vi "Dashboard Main.vi"() -> ()   [LabVIEW 2015]
uses:
  Vision FRC Color Processing Example Folder - Copy/Vision Support Code/Camera Types.ctl
  <vilib>/Utility/miscctls.llb/LVRowAndColumnTypeDef.ctl
  <vilib>/event_ctls.llb/eventvkey.ctl
  <vilib>/Rock Robotics/Network Tables/NT Write Boolean.vi
  <vilib>/Rock Robotics/Network Tables/NT Read Boolean.vi
  <vilib>/Rock Robotics/WPI/Dashboard/WPI_DashboardLogging Global.vi
  <vilib>/Utility/config.llb/Write Key (String).vi
  <vilib>/Utility/config.llb/Write Key (I32).vi
  <vilib>/Rock Robotics/Network Tables/NT Read Numeric Array.vi
  <vilib>/Utility/config.llb/NI_LVConfig.lvlib
panel:
  in  "Camera Type":T1=enum."1011"
  in  "TCP":refnum<k5>
  in  "Rec Mode":enum32{"Stop", "Record", "Playback"}(radio)
  in  "Vision":u16(ring) items=["Camera Off", "USB Camera SW", "USB Camera HW", "IP Camera"]
  out "Camera IP":string
  out "Image Message":string="Timeout in Camera Communications"
  in  "Dashboard Tab":T2(tab)=enum."Custom"
  out "Shooter Current":dbl(slide) scale=0.0..40.0
  out "Angle At Setpoint":bool=TRUE
  in  "Shoot":bool
  in  "Defense Type":T3(ring)
  out "NT Connection":bool
  in  "Camera Settings":T4={"Frame Rate"=30, "Compression"=30, "Size"=1} {"Frame Rate" scale=1.0..30.0; "Size" items=["640x480", "320x240", "160x120"]}
  out "Mode":T5(ring)=enum."Auto Disabled"
  in  "DB Camera Config":bool
  out "fps":dbl format="%#.1g"
  out "Mbps":dbl format="%#.1g"
  out "Mbps LED":bool
  out "Arm Encoder":dbl(slide) scale=-1.0..1.0
  out "At Target":bool
  in  "Defense Location":enum16{"0", "1", "2", "3", "4", "5"}(ring)
  in  "DB/String 0":string
  in  "DB/Slider 1":dbl(slide) scale=0.0..5.0
  out "DB/LED 1":bool
  out "DB/LED 0":bool
  in  "DB/Button 3":bool
  in  "DB/Button 2":bool
  in  "DB/Button 1":bool caption="LED Light"
  in  "DB/Button 0":bool
  out "JS1 Z":dbl(slide) scale=-1.0..1.0 scale format="%#_2e"
  out "JS1 Graph":cluster{"X":dbl, "Y":dbl}[](graph)
  out "JS1 Buttons":T6
  out "JS2 Z":dbl(slide) scale=-1.0..1.0 scale format="%#_2e"
  out "JS2 Graph":cluster{"X":dbl, "Y":dbl}[](graph)
  out "JS2 Buttons":T6
  out "Shooter Current":dbl(graph)
  out "Detected Targets":T7(array[cluster]) {"Normalized Rect"."Numeric 5" format="%#_2g"; "Normalized Rect"."Numeric 3" format="%#_2g"; "Normalized Rect"."Numeric 2" format="%#_2g"; "Normalized Rect"."Numeric" format="%#_2g"}
  in  "LED Color":T8={"Hue"={85.0, 140.0}, "Sat"={190.0, 255.0}, "Val"={70.0, 255.0}} {"Hue" scale=0.0..255.0 scale format="%#_3g"}
  in  "Std Devs for Calibration":cluster{"H":dbl, "S":dbl, "V":dbl}={"H"=4.0, "S"=6.0, "V"=6.0}
  in  "Min Score Threshold":i32=70
  out "Target Distance":dbl
  out "Target X":dbl
  out "Target Y":dbl
  in  "Test Slider":dbl(slide) scale=0.0..100.0 scale format="%#_3g"
  in  "On/Off":bool caption="Solenoid"
  in  "Test Name":u16(ring) items=["Select the test to run..."]
  in  "Test Tree":string(tree)
  in  "Motor":cluster{"Value":dbl, "Enable":bool} {"Value" scale=-1.0..1.0 scale format="%#_3g"}
  out "Progress":T9 {"Test Progress" scale=0.0..100.0}
  in  "Rev/Fwd":cluster{"Forward":bool, "Reverse":bool}
  in  "Test Ring":u16(ring) items=["Monochrome", "Color"]
  out "Cmd Status":string
  in  "Execute Command":bool
  in  "Command Params":string[][](table)
  in  "Command Selection":i32(listbox)
  in  "CheckList":i32(listbox)
  out "Tree":string(tree)
  out "Camera Image":T10(plugin-control)
  out "Background":bool
  # "Right"
  # "Left"
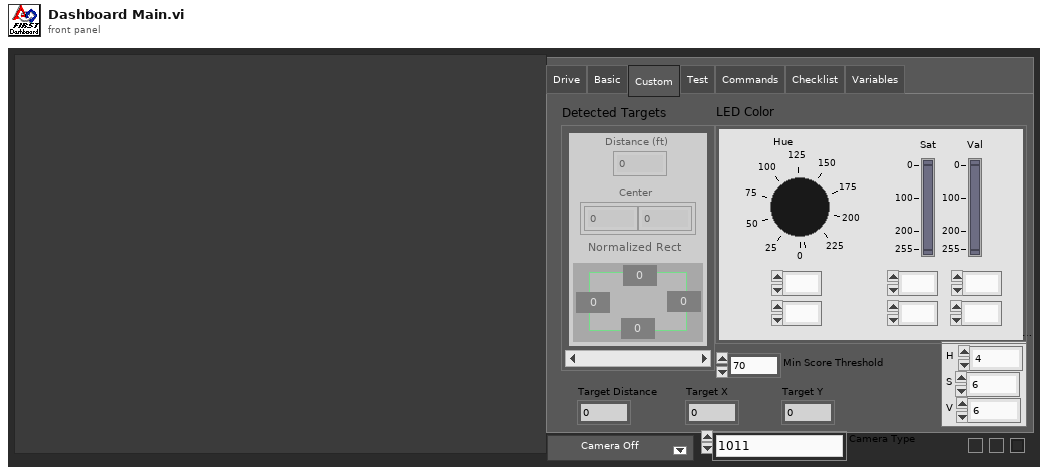
[diagram p1: front panel]
types:
  T1 = typedef "Camera Types.ctl" = enum16{"206", "1011", "1013", "MS HD3000 square", "MS HD3000 640x480"}
  T2 = enum32{"Drive", "Basic", "Custom", "Test", "Commands", "Checklist", "Variables"}
  T3 = enum16{"None", "Rampart", "Moat", "Rock Wall", "Rough Terrain", "Low Bar", "Chili Fries"}
  T4 = cluster{"Frame Rate":i32, "Compression":i32, "Size":u16}
  T5 = enum8{"Tele-Op Disabled", "Tele-Op Enabled", "Auto Disabled", "Auto Enabled", "Test Disabled", "Test Enabled", "Disconnected", "No Code", "E-Stop"}
  T6 = cluster{bool, bool, bool, bool, bool, bool, bool, bool, bool, bool, bool, bool}
  T7 = cluster{"Distance (ft)":dbl, "Center":cluster{dbl, dbl}, "Normalized Rect":cluster{"Numeric":dbl, "Numeric 2":dbl, "Numeric 3":dbl, "Numeric 5":dbl}}[]
  T8 = cluster{"Hue":cluster{dbl, dbl}, "Sat":cluster{dbl, dbl}, "Val":cluster{dbl, dbl}}
  T9 = cluster{"Test Progress":u8, "Test Progress Text":string}
  T10 = typedef "IMAQ Image.ctl" = refnum<image>
  T11 = cluster{"IDs":cluster{"RPC field ID":u16, "Unique ID":u16}, "String":string}
  T12 = enum32{"Drive", "Basic", "Custom", "Test", "Checklist", "Variables"}
  T13 = typedef "Image Type" = u32
  T14 = cluster{"Detected Targets[0]":cluster{"Distance (ft)":dbl, "Center":cluster{dbl, dbl}, "Normalized Rect":cluster{"Numeric":dbl, "Numeric 2":dbl, "Numeric 3":dbl, "Numeric 5":dbl}}, "Detected Targets[1]":cluster{"Distance (ft)":dbl, "Center":cluster{dbl, dbl}, "Normalized Rect":cluster{"Numeric":dbl, "Numeric 2":dbl, "Numeric 3":dbl, "Numeric 5":dbl}}, "Detected Targets[2]":cluster{"Distance (ft)":dbl, "Center":cluster{dbl, dbl}, "Normalized Rect":cluster{"Numeric":dbl, "Numeric 2":dbl, "Numeric 3":dbl, "Numeric 5":dbl}}, "Detected Targets[3]":cluster{"Distance (ft)":dbl, "Center":cluster{dbl, dbl}, "Normalized Rect":cluster{"Numeric":dbl, "Numeric 2":dbl, "Numeric 3":dbl, "Numeric 5":dbl}}, "Detected Targets[4]":cluster{"Distance (ft)":dbl, "Center":cluster{dbl, dbl}, "Normalized Rect":cluster{"Numeric":dbl, "Numeric 2":dbl, "Numeric 3":dbl, "Numeric 5":dbl}}, "Detected Targets[5]":cluster{"Distance (ft)":dbl, "Center":cluster{dbl, dbl}, "Normalized Rect":cluster{"Numeric":dbl, "Numeric 2":dbl, "Numeric 3":dbl, "Numeric 5":dbl}}, "Detected Targets[6]":cluster{"Distance (ft)":dbl, "Center":cluster{dbl, dbl}, "Normalized Rect":cluster{"Numeric":dbl, "Numeric 2":dbl, "Numeric 3":dbl, "Numeric 5":dbl}}, "Detected Targets[7]":cluster{"Distance (ft)":dbl, "Center":cluster{dbl, dbl}, "Normalized Rect":cluster{"Numeric":dbl, "Numeric 2":dbl, "Numeric 3":dbl, "Numeric 5":dbl}}, "Detected Targets[8]":cluster{"Distance (ft)":dbl, "Center":cluster{dbl, dbl}, "Normalized Rect":cluster{"Numeric":dbl, "Numeric 2":dbl, "Numeric 3":dbl, "Numeric 5":dbl}}}
  T15 = cluster{"Distance (ft)":dbl, "Center":cluster{dbl, dbl}, "Normalized Rect":cluster{"Numeric":dbl, "Numeric 2":dbl, "Numeric 3":dbl, "Numeric 5":dbl}}
  T16 = cluster{"Numeric":dbl, "Numeric 2":dbl, "Numeric 3":dbl, "Numeric 5":dbl}
  T17 = cluster{"Camera Image":refnum<vi>, "Dashboard Tab":refnum<vi>, "Background":refnum<vi>, "Vision":refnum<vi>, "Rec Mode":refnum<vi>, "Test Slider":refnum<vi>, "On/Off ":refnum<vi>, "Test Ring":refnum<vi>, "Rev/Fwd":refnum<vi>, "Test Name":refnum<vi>, "Motor":refnum<vi>, "Progress":refnum<vi>, "CheckList":refnum<vi>, "Tree":refnum<vi>, "Test Tree":refnum<vi>, "Command Params":refnum<vi>, "Command Selection":refnum<vi>, "Execute Command":refnum<vi>, "Cmd Status":refnum<vi>}
  T18 = typedef "NI_LVConfig.lvlib/Config Data RefNum.ctl" = refnum<k1>
  T19 = cluster{"Operation":enum16{"Update", "Clear"}, "Color Box":u32}[]
  T20 = typedef "eventvkey.ctl" = enum16{"ASCII", "Enter", "Return", "Shift", "Ctrl", "Alt", "Cmd", "Opt", "Caps", "NumLock", "Clear", "Break", "Up", "Down", "Left", "Right", "Insert", "Delete", "Home", "End", "PageUp", "PageDown", "Escape", "Help", "Pause", "ScrollLock", "F1", "F2", "F3", "F4", "F5", "F6", "F7", "F8", "F9", "F10", "F11", "F12", "F13", "F14", "F15", "F16", "F17", "F18", "F19", "F20", "F21", "F22", "F23", "F24", "Play", "VolumeUp", "VolumeDown", "Mute", "Two Byte Char"}
  T21 = cluster{"Image Size":bool, "Image Type":bool, "Pixel Value":bool, "ROI Information":bool, "Zoom Factor":bool}
  T22 = enum8{"Enabled", "Disabled", "Disabled and Grayed Out"}
  T23 = cluster{"Operation":enum16{"Update", "Clear"}, "Color Box":u32}
  T24 = typedef "LVRowAndColumnTypeDef.ctl" = cluster{"Row":i32, "Column":i32}
  T25 = cluster{"Shift":bool, "Ctrl":bool, "Alt":bool, "Cmd":bool, "Opt":bool}
  T26 = enum16{"open", "open or create", "create or replace", "create", "open (read only)"}
  T27 = cluster{"Error Strings":string, "Disable Counts":cluster{u16, u16}, "Rail Faults":cluster{u16, u16, u16}, "Robot IP":string, "DB Mode":u8, "Event Info":cluster{"Name":string, "Type":u8, "Number":u16, "Replay":u8}, "Camera Addr":string}
  T28 = cluster{"Storage":cluster{"Disk Free":u64, "RAM Block":u32, "RAM free":u32}, "CPU Utilization":cluster{"CPU % ISR":sgl, "CPU % Time Crit":sgl, "CPU % Timed Str":sgl, "CPU % High":sgl, "CPU % Above":sgl, "CPU % Normal":sgl, "CPU % Low":sgl}, "CAN":cluster{"% Bus Utilization":sgl, "Bus Off Cnt":u32, "TX_FIFO Full Cnt":u32, "Receive Error Cnt":u8, "Transmit Error Cnt":u8}, "HID":cluster{"HID Outputs":u32, "Rumble Low":u16, "Rumble High":u16}[]}
  T29 = cluster{"Status bits":cluster{"Test Mode":bool, "Autonomous":bool, "Enabled":bool, "Code Start":bool, "Brownout":bool, "Reserved 2":bool, "Reserved 3":bool, "E-Stop":bool}, "Code Trace":cluster{"Disabled":bool, "TeleOp":bool, "Auto":bool, "Test":bool}, "Controller Type":enum16{"unknown", "cRIO", "roboRio"}, "Code?":enum16{"unknown", "noCode", "code"}, "Battery V":dbl}
  T30 = cluster{"Control Bits":cluster{"TestMode":bool, "Autonomous":bool, "Enabled":bool, "FMS Present":bool, bool, bool, bool, "E-Stop":bool}, "Team Station ":u8, "Countdown":sgl, "Joystick Values":cluster{"Axes":dbl[], "Buttons":bool[], "POVs":i16[]}[]}
  T31 = cluster{"Axes":dbl[], "Buttons":bool[], "POVs":i16[]}[]
  T32 = cluster{"Test Mode":bool, "Autonomous":bool, "Enabled":bool, "Code Start":bool, "Brownout":bool, "Reserved 2":bool, "Reserved 3":bool, "E-Stop":bool}
  T33 = cluster{"Axes":dbl[], "Buttons":bool[], "POVs":i16[]}
  T34 = cluster{"Buttons[0]":bool, "Buttons[1]":bool, "Buttons[2]":bool, "Buttons[3]":bool, "Buttons[4]":bool, "Buttons[5]":bool, "Buttons[6]":bool, "Buttons[7]":bool, "Buttons[8]":bool, "Buttons[9]":bool, "Buttons[10]":bool, "Buttons[11]":bool}
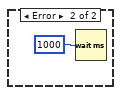
[diagram p2: hidden frame]
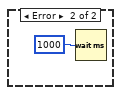
[diagram p3: hidden frame]
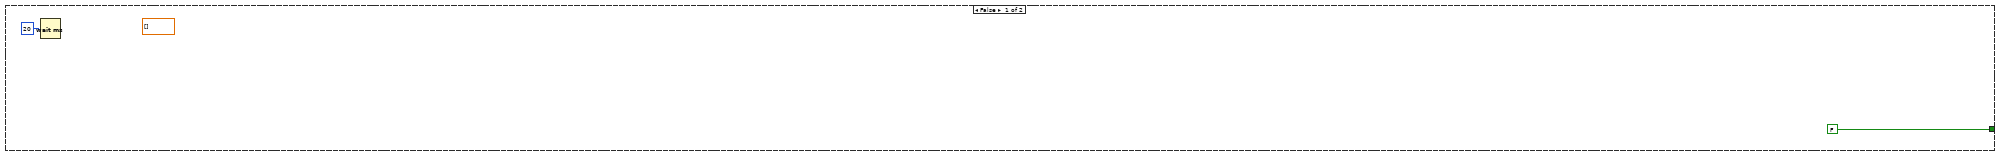
[diagram p4: hidden frame]
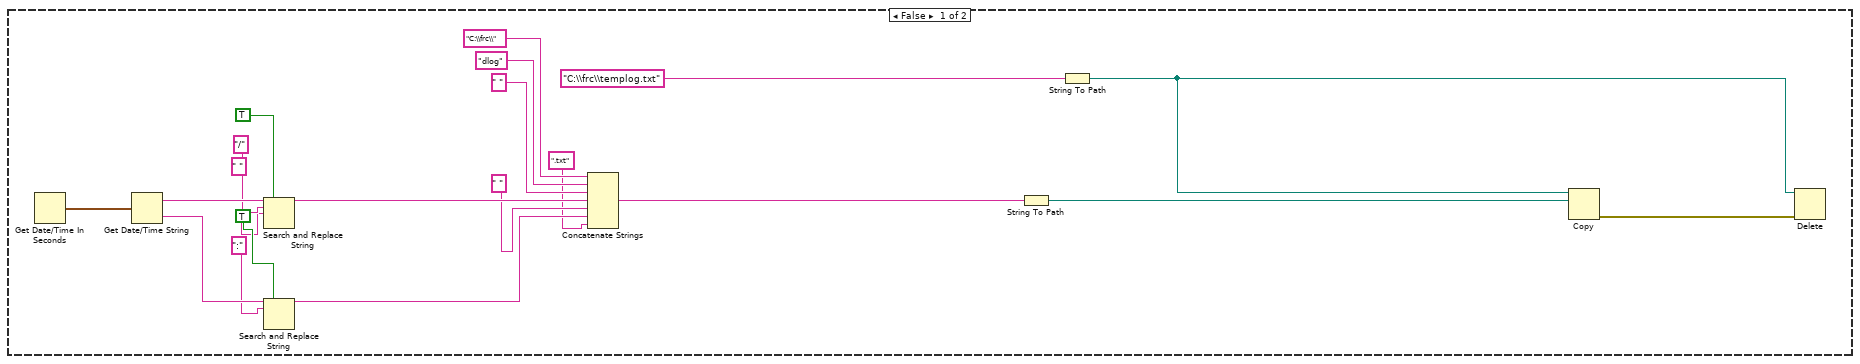
[diagram p5: hidden frame]
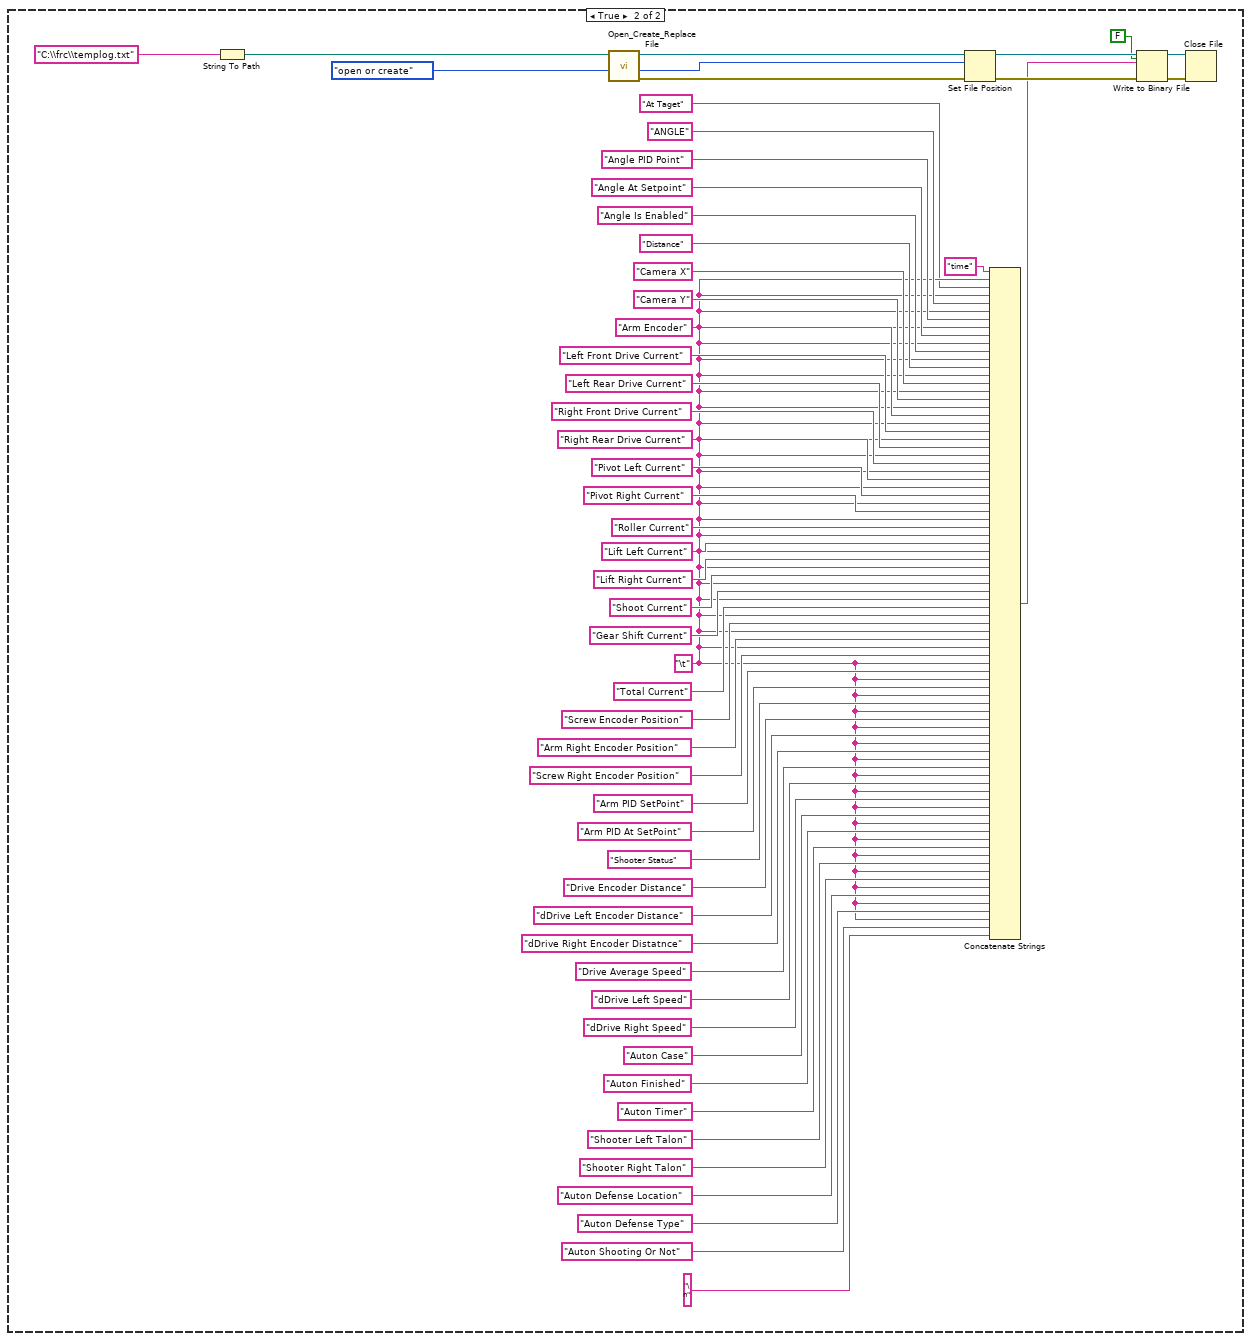
[diagram p6: hidden frame]
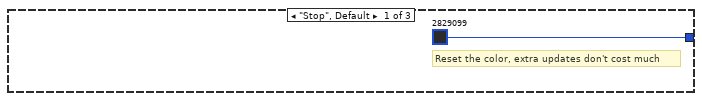
[diagram p7: hidden frame]
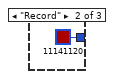
[diagram p8: hidden frame]
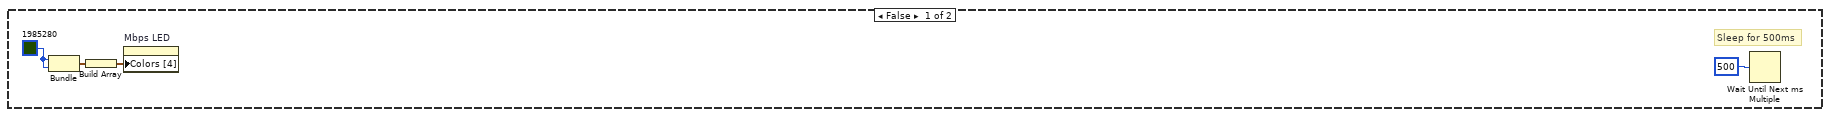
[diagram p10: hidden frame]
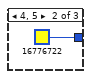
[diagram p11: hidden frame]
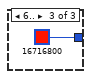
[diagram p12: hidden frame]
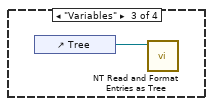
[diagram p14: hidden frame]
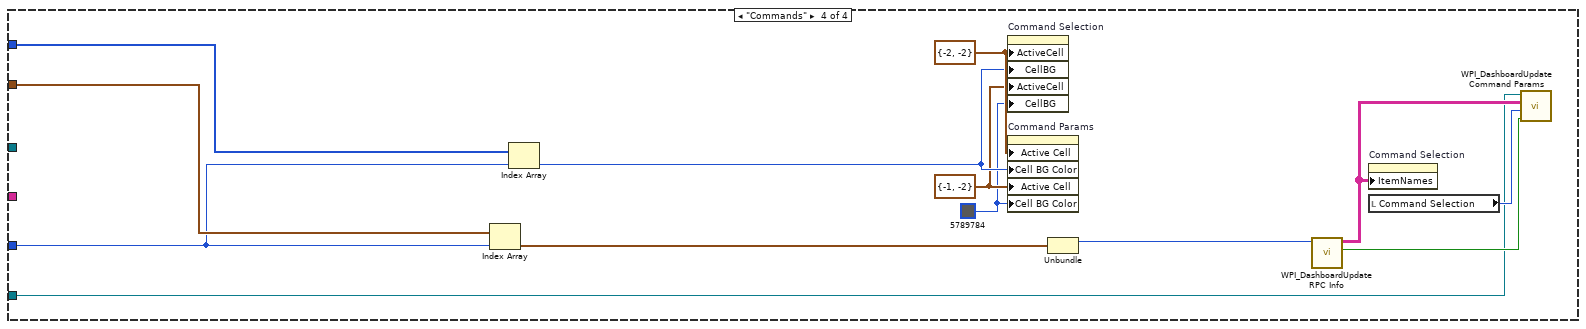
[diagram p15: hidden frame]
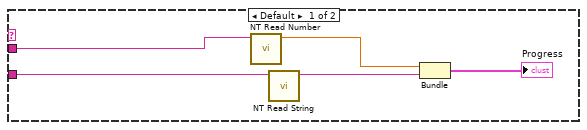
[diagram p16: hidden frame]
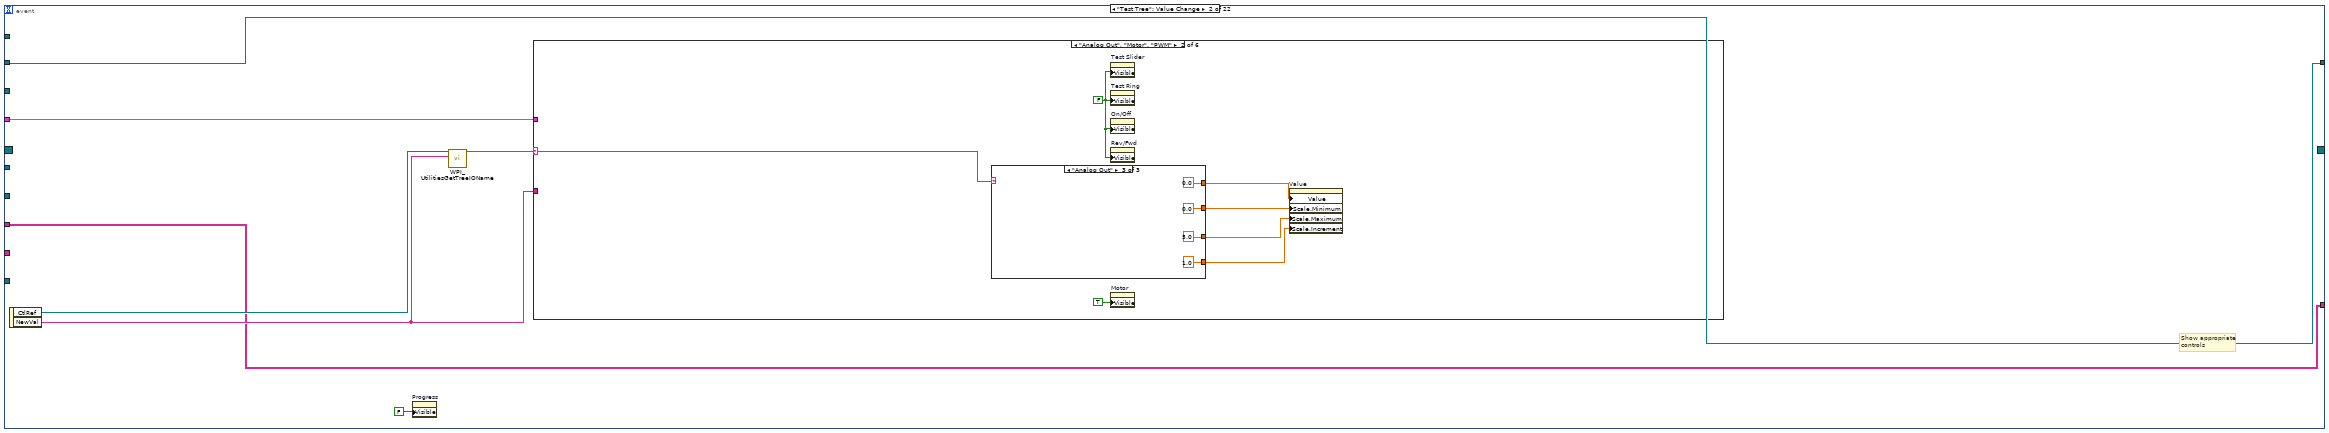
[diagram p17: hidden frame]
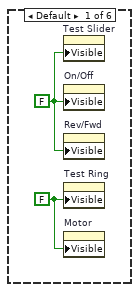
[diagram p18: hidden frame]
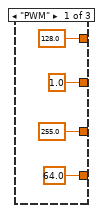
[diagram p19: hidden frame]
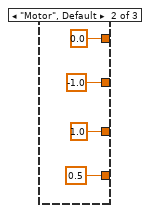
[diagram p20: hidden frame]
diagram:
  w10 = T11 {"IDs"={"RPC field ID"=0, "Unique ID"=0}, "String"=""}  # RPC Response
  w34 = 491  # min tab size
  w33 = 1.333  # min tab size
  w42 = enum32{"Stop", "Record", "Playback"}."Stop" ("Rec Mode")
  w16 = FALSE ("Visible")
  (unwired) "This VI has seven parallel loops for different tasks and a bit of initialization code that runs just once.\n\nTypical dashboard extensions only need to edit the panel. Adding new indicators or controls simply involves placing them on the panel in the Operations tab and naming them the same as the SmartDashboard variable on the robot\n\nIf the display needs to process the data before display, loop one is an example of doing that for the joysticks and motors.\n\nIf you want customize the video display or perform processing on it, loop two is where that takes place.\n\nOther loops should not need to be modified. They are pretty standard, and document the task they perform."  # Documentation
  w62 = T13 4 items=["Grayscale (U8)", "Grayscale (I16)", "Grayscale (SGL)", "Complex (CSG)", "RGB (U32)", "HSL (U32)", "RGB (U64)"] ("Image Type")
  # "Loop 7. Wait for DS connections"
  # "Controls for Test Mode, Camera Settings, etc."
  # "Loop 6. Animation for background of window during playback and record"
  # "Fires each time robot IP\nchanges, simulator does this"
  # "Fires each time window\ndocking changes."
  # "Collects all controls and indicators\nin the Basic and Custom tab.\nIf you need to bind additional controls,\nadd their references. You can extend the\nenum constant or use an integer."
  # "Loop 4. Process UI events related to test mode, checklist, and camera settings"
  # "Loop 3. Wait until the robot response provides\n the Robot IP address.\nOnce known, bind controls and\nvariables with the same names."
  # "Loop 5. Adjusts placement onscreen, hides the titlebar, etc."
  # "Loop 1. Receive various data streams from Driver Station, update joystick, motors, and more complex displays that don't easily bind to variables."
  # "Loop 2. Receive camera images from Robot, update Mbps, fps, and do any processing or display"
  n1 = control-ref of="Dashboard Tab"() -> (w40:refnum<vi>)
  n2 = property class="VI"() -> ("Panel"=w49:refnum<vi>)  [unwired: 2 in, 2 out]
  n3 = property on="Camera Settings" class="Clust (strict)"("Visible"=w16) -> ()  [unwired: 2 in, 2 out]
  n4 = property on="On/Off" class="Bool (strict)"("Visible"=w16) -> ()  [unwired: 2 in, 2 out]
  n5 = property on="Rev/Fwd" class="Clust (strict)"("Visible"=w16) -> ()  [unwired: 2 in, 2 out]
  n6 = local write "DB Camera Config"(w16) -> ()
  n7 = property on="Motor" class="Clust (strict)"("Visible"=w16) -> ()  [unwired: 2 in, 2 out]
  n8 = property on="Progress" class="Clust (strict)"("Visible"=w16) -> ()  [unwired: 2 in, 2 out]
  n9 = property on="Test Ring" class="Ring (strict)"("Visible"=w16) -> ()  [unwired: 2 in, 2 out]
  n10 = local write "Command Selection"(u16 0 ("milliseconds to wait")) -> ()
  n11 = local write "Rec Mode"(w42) -> ()
  n12 = global write "WPI_DashboardLogging Global.vi" "Recording"(w42) -> ()
  n13 = property class="Pnl"(reference=w49) -> ("Panes[]"=w50:refnum<vi>[])  [unwired: 1 in, 2 out]
  n14 = local write "Command Params"(string[][] [] ("Command Params")) -> ()
  n15 = local write "Dashboard Tab"(T2."Drive" ("Dashboard Tab")) -> ()
  n16 = call "IMAQ Create"("Image Name"="Dashboard Image", "Image Type"=w62) -> ("New Image"=w60:T10, "error out"=w59:errorcluster)  [unwired: 2 in, 1 out]
  n17 = Index Array(array=w50) -> (element=w48:refnum<vi>)  [unwired: 1 in]
  n18 = while {
    tunnel: w60 -> [w80]
    tunnel: w59 -> [_]
    tunnel: [w81] -> _
    i -> [w81]
    stop <- FALSE stop-if-true
    # "Optionally read the DB image,\nlog, or retrieve images from a\nlogged match"
    n19 = local read "Shooter Current"() -> (→"Shooter Current":dbl)
    n20 = call-poly <vilib>:"NT Write Value.vi"("Numeric"="Defense Type", "Name"="Defense Type") -> ()  [unwired: 9 in, 1 out]
    n21 = call-poly <vilib>:"NT Write Value.vi"("Numeric"="Defense Location", "Name"="Defense Location") -> ()  [unwired: 9 in, 1 out]
    n22 = call-poly <vilib>:"NT Read Value.vi"("Name"="Angle At Setpoint") -> ("Boolean"=→"Angle At Setpoint":bool)  [unwired: 9 in, 1 out]
    n23 = call-poly <vilib>:"NT Write Value.vi"("Boolean"="Shoot", "Name"="Shoot") -> ()  [unwired: 9 in, 1 out]
    n24 = local read "Camera IP"() -> (w74:string)
    n25 = local read "Rec Mode"() -> (w75:enum32{"Stop", "Record", "Playback"})
    n26 = call <vilib>:"WPI_CameraRead MJPG for Dashboard.vi"("Camera Settings"="Camera Settings", "Rec Mode"=w75, "Camera IP"=w74, "Camera Mode"="Vision", "Refnum in"=w80) -> ("Active"=w78:bool, "Refnum out"=w79:T10, "FPS"=w77:dbl, "Bandwidth (Mbps)"=w73:dbl)  [unwired: 3 in]
    "Mbps" <- w73
    n27 = case shown="True" w78 {
      tunnel: w79 -> [_ w177]
      tunnel: w73 -> [_ w176]
      tunnel: w77 -> [_ w175]
      frame False {
        w83 = u32 1985280 ("Color Box")
        # "Sleep for 500ms"
        n28 = Bundle("Color Box"=w83, "Color Box"=w83) -> (w85:cluster{"Color Box":u32, "Color Box":u32})  [unwired: 1 out]
        n29 = Build Array(w85) -> (w84:cluster{"Color Box":u32, "Color Box":u32}[])
        n30 = property on="Mbps LED" class="Bool (strict)"("Colors [4]"=w84) -> ()  [unwired: 2 in, 2 out]
        n31 = Wait Until Next ms Multiple(millisecond multiple=u32 500) -> ()  [unwired: 1 out]
      }
      frame True {
        # "Here is where you would annotate,\npossibly process, and display the image"
        # "Update Mbps LED"
        n32 = case shown="Default" w176 {
          tunnel: [u32 6618880 ("Color Box") u32 16776722 ("Color Box") u32 16716800 ("Color Box")] -> w178
          frame Default {
          }
          frame 4, 5 {
          }
          frame 6.. {
          }
        }
        n33 = call "IMAQ Clear Overlay"("Image"=w177) -> ("error out"=w181:errorcluster, "Image Out"=w174:T10)  [unwired: 2 in, 7 out]
        n34 = Unbundle By Name(w181) -> ("status"=w182:bool)
        n35 = call "FRC Color Processing Example.vi"("Std Devs for Calibration"="Std Devs for Calibration", "LED Color"="LED Color", "Min Score Threshold"="Min Score Threshold", "New Image"=w174, "Camera Type"="Camera Type") -> ("Detected Targets"=w131:T7, "Original Image"=→"Camera Image":T10)  [unwired: 5 in]
        "Detected Targets" <- w131
        n36 = property on="Image Message" class="Str"("Visible"=w182) -> ()  [unwired: 2 in, 2 out]
        n37 = Bundle("Color Box"=w178, "Color Box"=w178) -> (w180:cluster{"Color Box":u32, "Color Box":u32})  [unwired: 1 out]
        n38 = Array To Cluster(array=w131) -> (cluster=w169:T14)
        n39 = Build Array(w180) -> (w179:cluster{"Color Box":u32, "Color Box":u32}[])
        n40 = property on="Mbps LED" class="Bool (strict)"("Colors [4]"=w179) -> ()  [unwired: 2 in, 2 out]
        n41 = Unbundle(w169) -> ("Detected Targets[0]"=w168:T15, "Detected Targets[1]"=w144:T15, "Detected Targets[2]"=w132:T15)  [unwired: 6 out]
        n42 = Unbundle(w168) -> ("Distance (ft)"=w105:dbl, "Center"=w167:cluster{dbl, dbl}, "Normalized Rect"=w166:T16)
        n43 = Unbundle(w144) -> ("Distance (ft)"=w100:dbl, "Center"=w145:cluster{dbl, dbl}, "Normalized Rect"=w146:T16)
        n44 = Unbundle(w132) -> ("Distance (ft)"=w94:dbl, "Center"=w143:cluster{dbl, dbl}, "Normalized Rect"=w142:T16)
        n45 = Not Equal To 0?(x=w105) -> (x != 0?=w108:bool)
        n46 = Not Equal To 0?(x=w100) -> (x != 0?=w103:bool)
        n47 = Not Equal To 0?(x=w94) -> (x != 0?=w97:bool)
        n48 = Unbundle(w167) -> (w126:dbl)  [unwired: 1 out]
        n49 = Unbundle(w166) -> ("Numeric"=w158:dbl, "Numeric 2"=w125:dbl, "Numeric 3"=w156:dbl, "Numeric 5"=w160:dbl)
        n50 = Unbundle(w145) -> (w130:dbl)  [unwired: 1 out]
        n51 = Unbundle(w146) -> ("Numeric"=w153:dbl, "Numeric 2"=w124:dbl, "Numeric 3"=w155:dbl, "Numeric 5"=w151:dbl)
        n52 = Unbundle(w143) -> (w129:dbl)  [unwired: 1 out]
        n53 = Unbundle(w142) -> ("Numeric"=w135:dbl, "Numeric 2"=w123:dbl, "Numeric 3"=w133:dbl, "Numeric 5"=w137:dbl)
        n54 = Build Array(w126, w130, w129) -> (w127:dbl[])
        n55 = Build Array(w125, w124, w123) -> (w122:dbl[])
        n56 = Select(t=w105, s=w108, f=100.0) -> (s? t:f=w104:dbl)
        n57 = Select(t=w100, s=w103, f=100.0) -> (s? t:f=w99:dbl)
        n58 = Select(t=w94, s=w97, f=100.0) -> (s? t:f=w95:dbl)
        n59 = call-poly <vilib>:"NT Write Value.vi"("Numeric"=w126, "Name"="ImageXCenter0") -> ()  [unwired: 9 in, 1 out]
        n60 = call-poly <vilib>:"NT Write Value.vi"("Numeric"=w158, "Name"="ImageLeft0") -> ()  [unwired: 9 in, 1 out]
        n61 = call-poly <vilib>:"NT Write Value.vi"("Numeric"=w125, "Name"="ImageTop0") -> ()  [unwired: 9 in, 1 out]
        n62 = call-poly <vilib>:"NT Write Value.vi"("Numeric"=w156, "Name"="ImageRight0") -> ()  [unwired: 9 in, 1 out]
        n63 = call-poly <vilib>:"NT Write Value.vi"("Numeric"=w160, "Name"="ImageBottom0") -> ()  [unwired: 9 in, 1 out]
        n64 = call-poly <vilib>:"NT Write Value.vi"("Numeric"=w130, "Name"="ImageXCenter1") -> ()  [unwired: 9 in, 1 out]
        n65 = call-poly <vilib>:"NT Write Value.vi"("Numeric"=w153, "Name"="ImageLeft1") -> ()  [unwired: 9 in, 1 out]
        n66 = call-poly <vilib>:"NT Write Value.vi"("Numeric"=w124, "Name"="ImageTop1") -> ()  [unwired: 9 in, 1 out]
        n67 = call-poly <vilib>:"NT Write Value.vi"("Numeric"=w155, "Name"="ImageRight1") -> ()  [unwired: 9 in, 1 out]
        n68 = call-poly <vilib>:"NT Write Value.vi"("Numeric"=w151, "Name"="ImageBottom1") -> ()  [unwired: 9 in, 1 out]
        n69 = call-poly <vilib>:"NT Write Value.vi"("Numeric"=w129, "Name"="ImageXCenter2") -> ()  [unwired: 9 in, 1 out]
        n70 = call-poly <vilib>:"NT Write Value.vi"("Numeric"=w135, "Name"="ImageLeft2") -> ()  [unwired: 9 in, 1 out]
        n71 = call-poly <vilib>:"NT Write Value.vi"("Numeric"=w123, "Name"="ImageTop2") -> ()  [unwired: 9 in, 1 out]
        n72 = call-poly <vilib>:"NT Write Value.vi"("Numeric"=w133, "Name"="ImageRight2") -> ()  [unwired: 9 in, 1 out]
        n73 = call-poly <vilib>:"NT Write Value.vi"("Numeric"=w137, "Name"="ImageBottom2") -> ()  [unwired: 9 in, 1 out]
        n74 = Multiply(x=1.142, y=w104) -> (x*y=w110:dbl)
        n75 = Multiply(x=1.142, y=w99) -> (x*y=w116:dbl)
        n76 = Multiply(x=1.142, y=w95) -> (x*y=w113:dbl)
        n77 = Subtract(x=w110, y=1.0255) -> (x-y=w106:dbl)
        n78 = Subtract(x=w116, y=1.0255) -> (x-y=w101:dbl)
        n79 = Subtract(x=w113, y=1.0255) -> (x-y=w98:dbl)
        n80 = Build Array(w106, w101, w98) -> (w128:dbl[])
        n81 = call-poly <vilib>:"NT Write Value.vi"("Numeric"=w106, "Name"="distanceToTarget0") -> ()  [unwired: 9 in, 1 out]
        n82 = call-poly <vilib>:"NT Write Value.vi"("Numeric"=w101, "Name"="distanceToTarget1") -> ()  [unwired: 9 in, 1 out]
        n83 = call-poly <vilib>:"NT Write Value.vi"("Numeric"=w98, "Name"="distanceToTarget2") -> ()  [unwired: 9 in, 1 out]
        n84 = Array Max & Min(array=w128) -> (min value=w89:dbl, min index (indices)=w121:i32)  [unwired: 2 out]
        "Target Distance" <- w89
        n85 = Index Array(array=w127, index=w121) -> (element=w120:dbl)
        "Target X" <- w120
        n86 = Index Array(array=w122, index=w121) -> (element=→"Target Y":dbl)
        n87 = In Range and Coerce(upper limit=-0.1525, x=w120, lower limit=-0.1725) -> (In Range?=w91:bool)  [unwired: 1 out]
        n88 = Less?(x=w89, y=15.0) -> (x < y?=w90:bool)
        n89 = And(x=w91, y=w90) -> (x .and. y?=w88:bool)
        "At Target" <- w88
        n90 = call-poly <vilib>:"NT Write Value.vi"("Boolean"=w88, "Name"="At Target") -> ()  [unwired: 9 in, 1 out]
        "fps" <- w175
      }
    }
  }
  n91 = while {
    tunnel: u16 1741 ("timeout ms (25000)") -> [w187]
    stop <- FALSE stop-if-true
    n92 = TCP Create Listener(10:w187) -> (0:w186:errorcluster, 3:w188:refnum<k5>)  [unwired: 4 in, 1 out]
    n93 = case shown="No Error" w186 {
      selector: w186 -> [w190 _]
      tunnel: w188 -> [w191 _]
      frame No Error {
        n94 = while {
          tunnel: w191 -> [w194]
          tunnel: w190 -> [w193]
          stop <- FALSE stop-if-true
          n95 = TCP Wait On Listener(8:w193, 11:w194) -> (0:w195:errorcluster, 4:w196:refnum<k5>)  [unwired: 2 in, 3 out]
          n96 = case shown="No Error" w195 {
            frame No Error {
            }
            frame Error {
              n97 = Wait (ms)(milliseconds to wait=u32 1000) -> ()  [unwired: 1 out]
            }
          }
          n98 = local write "TCP"(w196) -> ()
        }
      }
      frame Error {
        n99 = Wait (ms)(milliseconds to wait=u32 1000) -> ()  [unwired: 1 out]
      }
    }
  }
  n100 = call <vilib>:"Get Tab Control Refs.vi"("Page Index"=T12."Custom" ("Dashboard Tab"), "TabControl in"=w40) -> ("ControlsOnPage"=w39:refnum<vi>[])  [unwired: 9 in]
  n101 = while {
    tunnel: w48 -> [w200]
    i -> [w203]
    stop <- FALSE stop-if-true
    n102 = case shown="\"Playback\"" "Rec Mode" {
      tunnel: w203 -> [_ _ w218]
      tunnel: [u32 2829099 ("Base Color") u32 11141120 ("Target Color") w207] -> w199
      frame "Stop", Default {
        # "Reset the color, extra updates don't cost much"
      }
      frame "Record" {
      }
      frame "Playback" {
        # "Playback"
        n103 = Quotient & Remainder(x=w218, y=u32 50 ("milliseconds to wait")) -> (x-y*floor(x/y)=w214:u32)  [unwired: 1 out]
        n104 = Divide(x=w214, y=u32 50 ("milliseconds to wait")) -> (x/y=w211:dbl)
        n105 = Multiply(x=6.283185307179586, y=w211) -> (x*y=w216:dbl)
        n106 = Sine(x=w216) -> (sin(x)=w215:dbl)
        n107 = Absolute Value(x=w215) -> (abs(x)=w208:dbl)
        n108 = call "Interpolate RGB Color.vi"("Proportion"=w208, "Target Color"=u32 30976, "Base Color"=u32 2829099) -> ("Result Color"=w207:u32)  [unwired: 8 in]
      }
    }
    n109 = Wait (ms)(milliseconds to wait=u32 100) -> ()  [unwired: 1 out]
    n110 = property class="Pane"(reference=w200, "PaneColor"=w199) -> ()  [unwired: 1 in, 2 out]
  }
  n111 = call <vilib>:"Get Tab Control Refs.vi"("Page Index"=T12."Basic" ("Dashboard Tab"), "TabControl in"=w40) -> ("ControlsOnPage"=w15:refnum<vi>[])  [unwired: 9 in]
  n112 = Build Array (concatenate)(w15, w39) -> (w38:refnum<vi>[])
  n113 = Obtain Notifier(name (unnamed)="Robot IP Update", notification data type="IP Addr" ("name (unnamed)")) -> (notifier out=w2:refnum<notifier>)  [unwired: 2 in, 2 out]
  n114 = Create User Event(user event datatype=w10) -> (user event=w6:refnum<user-event>)  [unwired: 1 in, 1 out]
  n115 = control-ref of="Rec Mode"() -> (w22:refnum<vi>)
  n116 = control-ref of="Command Selection"() -> (w9:refnum<vi>)
  n117 = control-ref of="Execute Command"() -> (w11:refnum<vi>)
  n118 = control-ref of="Command Params"() -> (w12:refnum<vi>)
  n119 = control-ref of="Camera Image"() -> (w37:refnum<vi>)
  n120 = control-ref of="Dashboard Tab"() -> (w36:refnum<vi>)
  n121 = control-ref of="Tree"() -> (w26:refnum<vi>)
  n122 = control-ref of="Test Tree"() -> (w25:refnum<vi>)
  n123 = control-ref of="Background"() -> (w31:refnum<vi>)
  n124 = control-ref of="Cmd Status"() -> (w5:refnum<vi>)
  n125 = control-ref of="On/Off"() -> (w20:refnum<vi>)
  n126 = control-ref of="Test Name"() -> (w24:refnum<vi>)
  n127 = control-ref of="Test Slider"() -> (w21:refnum<vi>)
  n128 = control-ref of="Rev/Fwd"() -> (w18:refnum<vi>)
  n129 = control-ref of="Motor"() -> (w23:refnum<vi>)
  n130 = control-ref of="Progress"() -> (w17:refnum<vi>)
  n131 = control-ref of="CheckList"() -> (w27:refnum<vi>)
  n132 = control-ref of="Test Ring"() -> (w19:refnum<vi>)
  n133 = control-ref of="Vision"() -> (w35:refnum<vi>)
  n134 = while {
    tunnel: w38 -> [w231]
    tunnel: w2 -> [w229]
    tunnel: [w227] -> _
    tunnel: u32 1000 ("milliseconds to wait") -> [w226]
    tunnel: w6 -> [w219]
    i -> [w227]
    stop <- FALSE stop-if-true
    n135 = Wait on Notification(notifier=w229, timeout in ms (-1)=w226) -> (notification=w228:string, timed out?=w224:bool)  [unwired: 2 in, 2 out]
    n136 = local read "Rec Mode"() -> (w222:enum32{"Stop", "Record", "Playback"})
    n137 = Equal?(x=w222, y=u16 2 ("Rec Mode")) -> (x = y?=w223:bool)
    n138 = Compound Arithmetic op=OR(invert w224, w223) -> (w225:bool)
    n139 = case shown="True" w225 {
      tunnel: w231 -> [_ w235]
      tunnel: w228 -> [_ w234]
      tunnel: "Dashboard" -> [_ w233]
      tunnel: w219 -> [_ w232]
      frame False {
      }
      frame True {
        n140 = call <vilib>:"Bind Controls to SmartDashboard.vi"("RPC ref"=w232, "Client Name"=w233, "Bound Control Refs"=w235, "Server IP Address"=w234) -> ()  [unwired: 8 in]
      }
    }
  }
  n141 = Bundle("Camera Image"=w37, "Dashboard Tab"=w36, "Background"=w31, "Vision"=w35, "Rec Mode"=w22, "Test Slider"=w21, "On/Off"=w20, "Test Ring"=w19, "Rev/Fwd"=w18, "Test Name"=w24, "Motor"=w23, "Progress"=w17, "CheckList"=w27, "Tree"=w26, "Test Tree"=w25, "Command Params"=w12, "Command Selection"=w9, "Execute Command"=w11, "Cmd Status"=w5) -> (w28:T17)  [unwired: 1 in]
  n142 = register-events(refnum<vi> refnum, w6) -> (reference out=w46:refnum<event-registration>, error out=w45:errorcluster)  [unwired: 2 in]
  n143 = call "Initialize Camera and CheckList.vi"("ListBox in"=w27) -> ("Cluster"=w53:cluster{"value":i32, "value":i32, "index":i32}, "Array"=w54:cluster{string[]}[], "File Refnum"=w52:T18)  [unwired: 8 in]
  n144 = property on="Camera Settings" class="Clust (strict)"("Val(Sgnl)"=w53) -> ()  [unwired: 2 in, 2 out]
  n145 = Bundle("min tab size"=w34, "min tab size"=w33) -> (w32:cluster{"min tab size":i32, "min tab size":dbl})  [unwired: 1 in]
  n146 = Obtain Notifier(name (unnamed)="Window Mode", notification data type=TRUE) -> (notifier out=w3:refnum<notifier>)  [unwired: 2 in, 2 out]
  n147 = vi-ref "Playback Controls.vi"() -> (w47:refnum<vi>)
  n148 = control-ref of="Command Params"() -> (w4:refnum<vi>)
  n149 = control-ref of="Test Tree"() -> (w51:refnum<vi>)
  n150 = property class="VI" props=["Front Panel.Closeable"]() -> (reference out=w41:refnum<vi>)  [unwired: 2 in, 2 out]
  n151 = call "Adjust Dashboard Window.vi"("Sizing Refnums"=w28, "Size Constraints"=w32, "VI"=w41, "WIn Mode"=w3) -> ()  [unwired: 8 in]
  n152 = while {
    tunnel: w54 -> [w247]
    shift-right: [w246] -> _
    shift-left: w52 -> [w245]
    tunnel: [w244] -> _
    tunnel: w51 -> [w243]
    tunnel: w47 -> [w242]
    tunnel: w46 -> [w241]
    tunnel: w45 -> [_]
    tunnel: w41 -> [w240]
    tunnel: w6 -> [w239]
    tunnel: w4 -> [w238]
    shift-right: [w237] -> _
    shift-left: _ -> [w236]
    i -> [w244]
    stop <- FALSE stop-if-true
    n153 = event shown="[0] Timeout" {
      selector: w241 -> [_ _ _ _ _ _ _ _ _ _ _ _ _ _ _ _ _ _ _ _ _ _]
      dyn-events: [_ _ _ _ _ _ _ _ _ _ _ _ _ _ _ _ w548 _ _ _ _ _] -> _
      timeout: u32 60 ("milliseconds to wait") -> [_ _ _ _ _ _ _ _ _ _ _ _ _ _ _ _ _ _ _ _ _ _]
      tunnel: w243 -> [w260 _ _ _ _ _ _ _ _ _ _ _ _ _ _ _ _ _ _ _ _ _]
      tunnel: "Test Tree" -> [_ _ _ _ _ _ _ _ _ _ _ w511 w520 w523 w528 w537 _ _ _ _ _ _]
      tunnel: w247 -> [_ w298 _ _ _ _ _ _ _ w473 w504 _ _ _ _ _ _ _ _ _ _ _]
      tunnel: [w257 w297 w401 w407 w419 w431 w439 w445 w458 w472 w497 w510 w518 w522 w527 w536 w550 w566 w568 w576 w587 w592] -> w246
      tunnel: w245 -> [w257 w297 w401 w407 w419 w431 w439 w445 w458 w471 w497 w510 w518 w522 w527 w536 w550 w566 w568 w576 w587 w592]
      tunnel: w242 -> [_ _ _ _ _ _ _ _ _ _ _ _ _ _ _ _ w551 _ w571 _ _ _]
      tunnel: w240 -> [_ _ _ _ _ _ _ _ _ _ _ _ _ _ _ _ w546 _ _ _ _ _]
      tunnel: w239 -> [_ _ _ _ _ _ _ _ _ _ _ _ _ _ _ _ w542 _ _ _ _ _]
      tunnel: w238 -> [w252 _ _ _ w417 _ _ _ _ _ _ _ _ _ _ _ _ _ _ _ _ _]
      tunnel: [w251 w296 w400 w406 w415 w425 w436 w444 w457 w470 w496 w509 w517 w521 w526 w535 w541 w564 w567 w572 w580 w593] -> w237
      tunnel: w236 -> [w251 w296 w400 w406 w415 _ _ w444 w457 w470 w496 w509 w517 w521 w526 w535 w541 w564 w567 w572 w580 w593]
      event Timeout {
        n154 = event-data() -> ()  [unwired: 1 in, 1 out]
        n155 = local read "Mode"() -> (w254:T5)
        n156 = call <vilib>:"Connextion Info.vi"() -> ("Connected"=→"NT Connection":bool)  [unwired: 10 in, 1 out]
        n157 = case shown="\"Test\"" "Dashboard Tab" {
          tunnel: w260 -> [_ w274 _ _]
          tunnel: "/TestMode/Automatic/" ("Name Pattern") -> [_ w273 _ _]
          tunnel: T19 [{"Operation"=enum."Clear", "Color Box"=14013909}, {"Operation"=enum."Clear", "Color Box"=14013909}, {"Operation"=enum."Clear", "Color Box"=14013909}, {"Operation"=enum."Clear", "Color Box"=14013909}, {"Operation"=enum."Update", "Color Box"=14013909}, {"Operation"=enum."Update", "Color Box"=16777215}, {"Operation"=enum."Clear", "Color Box"=14013909}, {"Operation"=enum."Clear", "Color Box"=14013909}, {"Operation"=enum."Clear", "Color Box"=14013909}] -> [_ w266 _ w283]
          tunnel: w254 -> [_ w265 _ w282]
          tunnel: u32[] [15790320, 15790320, 15790320, 15790320, 16777215, 16777215, 15790320, 15790320, 15790320] -> [_ _ _ w288]
          tunnel: w252 -> [_ _ _ w276]
          frame "Custom", Default {
          }
          frame "Test" {
            w272 = -2 ("Active Item:Row Number")
            n158 = Index Array(array=w266, index=w265) -> (element=w267:T23)
            n159 = Unbundle(w267) -> ("Operation"=w268:enum16{"Update", "Clear"}, "Color Box"=w269:u32)
            n160 = call <vilib>:"NT Read and Format Entries as Tree.vi"("Operation"=w268, "Name Pattern"=w273, "Tree Refnum"=w274) -> ()  [unwired: 7 in, 2 out]
            n161 = property on="Test Tree" class="Tree (strict)"("Active Item Row Number"=w272, "ActiveColNum"=w272, "CellBG"=w269, "Active Item Row Number"=-1 ("Active Item:Row Number"), "CellBG"=u32 5789784 ("Color Box")) -> ()  [unwired: 2 in, 2 out]
          }
          frame "Variables" {
            n162 = control-ref of="Tree"() -> (w275:refnum<vi>)
            n163 = call <vilib>:"NT Read and Format Entries as Tree.vi"("Tree Refnum"=w275) -> ()  [unwired: 9 in, 2 out]
          }
          frame "Commands" {
            w284 = u32 5789784 ("Color Box")
            w285 = T24 {"Row"=-1, "Column"=-2} ("Active Cell:Active Cell")
            w287 = T24 {"Row"=-2, "Column"=-2} ("Active Cell:Active Cell")
            n164 = Index Array(array=w283, index=w282) -> (element=w281:T23)
            n165 = Index Array(array=w288, index=w282) -> (element=w286:u32)
            n166 = property on="Command Selection" class="MCListbox (strict)"("ActiveCell"=w287, "CellBG"=w286, "ActiveCell"=w285, "CellBG"=w284) -> ()  [unwired: 2 in, 2 out]
            n167 = property on="Command Params" class="Tbl (strict)"("Active Cell"=w287, "Cell BG Color"=w286, "Active Cell"=w285, "Cell BG Color"=w284) -> ()  [unwired: 2 in, 2 out]
            n168 = Unbundle(w281) -> ("Operation"=w280:enum16{"Update", "Clear"})  [unwired: 1 out]
            n169 = call <vilib>:"WPI_DashboardUpdate RPC Info.vi"("Operation"=w280) -> ("update"=w278:bool, "commands"=w277:string[][])  [unwired: 9 in]
            n170 = property on="Command Selection" class="MCListbox (strict)"("ItemNames"=w277) -> ()  [unwired: 2 in, 2 out]
            n171 = local read "Command Selection"() -> (w279:i32)
            n172 = call <vilib>:"WPI_DashboardUpdate Command Params.vi"("Update"=w278, "NewVal"=w279, "Commands"=w277, "Param Tbl"=w276) -> ()  [unwired: 7 in, 1 out]
          }
        }
        n173 = call <vilib>:"NT Read String.vi"("Name"="/TestMode/TestName") -> ("String"=w263:string)  [unwired: 9 in, 1 out]
        n174 = case shown="\"\"" w263 {
          tunnel: "/TestMode/TestProgress" ("Name") -> [w290 _]
          tunnel: "/TestMode/TestProgressText" ("Name") -> [w289 _]
          frame Default {
            n175 = call <vilib>:"NT Read Number.vi"("Name"=w290) -> ("Numeric"=w291:dbl)  [unwired: 9 in, 1 out]
            n176 = call <vilib>:"NT Read String.vi"("Name"=w289) -> ("String"=w292:string)  [unwired: 9 in, 1 out]
            n177 = Bundle("Numeric"=w291, "String"=w292) -> (→"Progress":cluster{"Numeric":dbl, "String":string})  [unwired: 1 in]
          }
          frame "" {
            n178 = property on="Progress" class="Clust (strict)"("Visible"=FALSE) -> ()  [unwired: 2 in, 2 out]
            n179 = local write "Test Name"(u16 0) -> ()
          }
        }
      }
      event "Test Tree": Value Change {
        # "Show appropriate\ncontrols"
        n180 = event-data() -> ("CtlRef"=w301:refnum<vi>, "NewVal"=w299:string)  [unwired: 1 in]
        n181 = property on="Progress" class="Clust (strict)"("Visible"=FALSE) -> ()  [unwired: 2 in, 2 out]
        n182 = call <vilib>:"WPI_UtilitiesGetTreeIOName.vi"("NewVal"=w299, "TreeControl in"=w301) -> ("I/O Name"=w302:string)  [unwired: 9 in]
        n183 = case shown="\"Analog Out\", \"Motor\", \"PWM\"" w302 {
          selector: w302 -> [_ w309 _ w331 w340 _]
          tunnel: w299 -> [_ _ w328 w330 _ w347]
          tunnel: w298 -> [_ _ _ _ _ w346]
          frame Default {
            w304 = FALSE ("Visible")
            w303 = FALSE ("Visible")
            n184 = property on="Test Slider" class="Slide (strict)"("Visible"=w304) -> ()  [unwired: 2 in, 2 out]
            n185 = property on="On/Off" class="Bool (strict)"("Visible"=w304) -> ()  [unwired: 2 in, 2 out]
            n186 = property on="Rev/Fwd" class="Clust (strict)"("Visible"=w304) -> ()  [unwired: 2 in, 2 out]
            n187 = property on="Test Ring" class="Ring (strict)"("Visible"=w303) -> ()  [unwired: 2 in, 2 out]
            n188 = property on="Motor" class="Clust (strict)"("Visible"=w303) -> ()  [unwired: 2 in, 2 out]
          }
          frame "Analog Out", "Motor", "PWM" {
            w310 = FALSE ("Visible")
            n189 = case shown="\"Analog Out\"" w309 {
              tunnel: [1.0 ("Value") -1.0 ("Value") 0.0 ("Value")] -> w308
              tunnel: [255.0 ("Value") 1.0 ("Value") 5.0 ("Value")] -> w307
              tunnel: [128.0 ("Value") 0.0 ("Value") 0.0 ("Value")] -> w306
              tunnel: [64.0 ("Value") 0.5 ("Value") 1.0 ("Value")] -> w305
              frame "PWM" {
              }
              frame "Motor", Default {
              }
              frame "Analog Out" {
              }
            }
            n190 = property on="Test Slider" class="Slide (strict)"("Visible"=w310) -> ()  [unwired: 2 in, 2 out]
            n191 = property on="Test Ring" class="Ring (strict)"("Visible"=w310) -> ()  [unwired: 2 in, 2 out]
            n192 = property on="On/Off" class="Bool (strict)"("Visible"=w310) -> ()  [unwired: 2 in, 2 out]
            n193 = property on="Rev/Fwd" class="Clust (strict)"("Visible"=w310) -> ()  [unwired: 2 in, 2 out]
            n194 = property on="Motor" class="Clust (strict)"("Visible"=TRUE) -> ()  [unwired: 2 in, 2 out]
            n195 = property on="Value" class="Slide (strict)"("Value"=w306, "Scale.Minimum"=w308, "Scale.Maximum"=w307, "Scale.Increment"=w305) -> ()  [unwired: 2 in, 2 out]
          }
          frame "Servo" {
            w326 = FALSE ("Visible")
            n196 = call <vilib>:"NT Read Number.vi"("Name"=w328) -> ("Numeric"=w327:dbl)  [unwired: 9 in, 1 out]
            n197 = property on="Motor" class="Clust (strict)"("Visible"=w326) -> ()  [unwired: 2 in, 2 out]
            n198 = property on="Test Ring" class="Ring (strict)"("Visible"=w326) -> ()  [unwired: 2 in, 2 out]
            n199 = property on="On/Off" class="Bool (strict)"("Visible"=w326) -> ()  [unwired: 2 in, 2 out]
            n200 = property on="Rev/Fwd" class="Clust (strict)"("Visible"=w326) -> ()  [unwired: 2 in, 2 out]
            n201 = property on="Test Slider" class="Slide (strict)"("Visible"=TRUE, "Scale.Maximum"=170.0 ("Scale.Range:Maximum")) -> ()  [unwired: 2 in, 2 out]
            n202 = local write "Test Slider"(w327) -> ()
          }
          frame "Relay", "Solenoid" {
            w329 = FALSE ("Visible")
            n203 = property on="Motor" class="Clust (strict)"("Visible"=w329) -> ()  [unwired: 2 in, 2 out]
            n204 = property on="Test Slider" class="Slide (strict)"("Visible"=w329) -> ()  [unwired: 2 in, 2 out]
            n205 = property on="Test Ring" class="Ring (strict)"("Visible"=w329) -> ()  [unwired: 2 in, 2 out]
            n206 = Search and Replace String(input string=w330, search string="/Value  **", replace string="/Direction") -> (result string=w336:string)  [unwired: 5 in, 3 out]
            n207 = call <vilib>:"NT Read String.vi"("Name"=w336) -> ("String"=w334:string)  [unwired: 9 in, 1 out]
            n208 = Equal?(x="Both directions", y=w334) -> (x = y?=w332:bool)
            n209 = property on="Rev/Fwd" class="Clust (strict)"("Visible"=w332) -> ()  [unwired: 2 in, 2 out]
            n210 = Not(x=w332) -> (.not. x?=w333:bool)
            n211 = property on="On/Off" class="Bool (strict)"("Visible"=w333, "Caption.Text"=w331) -> ()  [unwired: 2 in, 2 out]
          }
          frame "Compressor", "Digital Out" {
            w339 = FALSE ("Visible")
            # "Get direction and finish"
            n212 = property on="Test Ring" class="Ring (strict)"("Visible"=w339) -> ()  [unwired: 2 in, 2 out]
            n213 = property on="Motor" class="Clust (strict)"("Visible"=w339) -> ()  [unwired: 2 in, 2 out]
            n214 = property on="Test Slider" class="Slide (strict)"("Visible"=w339) -> ()  [unwired: 2 in, 2 out]
            n215 = property on="Rev/Fwd" class="Clust (strict)"("Visible"=FALSE) -> ()  [unwired: 2 in, 2 out]
            n216 = property on="On/Off" class="Bool (strict)"("Visible"=TRUE, "Caption.Text"=w340) -> ()  [unwired: 2 in, 2 out]
          }
          frame "Camera" {
            n217 = call <vilib>:"Get Last Path Segment.vi"("String in"=w347) -> ("String out"=w348:string)  [unwired: 10 in]
            n218 = property on="Rev/Fwd" class="Clust (strict)"("Visible"=FALSE) -> ()  [unwired: 2 in, 2 out]
            n219 = case shown="\"White Balance  **\"" w348 {
              tunnel: w347 -> [w354 w363 w372 w381 w390 _ w396]
              tunnel: w346 -> [w352 w360 w369 w378 w387 _ _]
              frame "Size  **" {
                n220 = Index Array(array=w352) -> (element=w351:cluster{string[]})  [unwired: 1 in]
                n221 = call <vilib>:"NT Read String.vi"("Name"=w354) -> ("String"=w353:string)  [unwired: 9 in, 1 out]
                n222 = property on="Test Ring" class="Ring (strict)"("Visible"=TRUE) -> ()  [unwired: 2 in, 2 out]
                n223 = property on="Test Slider" class="Slide (strict)"("Visible"=FALSE) -> ()  [unwired: 2 in, 2 out]
                n224 = Unbundle(w351) -> (w349:string[])
                n225 = Match First String(2:w349, 3:w353) -> (0:w350:i32)  [unwired: 1 out]
                n226 = property on="Test Ring" class="Ring (strict)"("Value"=w350, "Strings []"=w349) -> ()  [unwired: 2 in, 2 out]
              }
              frame "White Balance  **" {
                n227 = call <vilib>:"NT Read String.vi"("Name"=w363) -> ("String"=w362:string)  [unwired: 9 in, 1 out]
                n228 = Index Array(array=w360, index=1) -> (element=w361:cluster{string[]})
                n229 = property on="Test Ring" class="Ring (strict)"("Visible"=TRUE) -> ()  [unwired: 2 in, 2 out]
                n230 = property on="Test Slider" class="Slide (strict)"("Visible"=FALSE) -> ()  [unwired: 2 in, 2 out]
                n231 = Unbundle(w361) -> (w358:string[])
                n232 = Match First String(2:w358, 3:w362) -> (0:w357:i32)  [unwired: 1 out]
                n233 = property on="Test Ring" class="Ring (strict)"("Value"=w357, "Strings []"=w358) -> ()  [unwired: 2 in, 2 out]
              }
              frame "Exposure  **" {
                n234 = call <vilib>:"NT Read String.vi"("Name"=w372) -> ("String"=w371:string)  [unwired: 9 in, 1 out]
                n235 = Index Array(array=w369, index=2) -> (element=w370:cluster{string[]})
                n236 = property on="Test Ring" class="Ring (strict)"("Visible"=TRUE) -> ()  [unwired: 2 in, 2 out]
                n237 = property on="Test Slider" class="Slide (strict)"("Visible"=FALSE) -> ()  [unwired: 2 in, 2 out]
                n238 = Unbundle(w370) -> (w366:string[])
                n239 = Match First String(2:w366, 3:w371) -> (0:w367:i32)  [unwired: 1 out]
                n240 = property on="Test Ring" class="Ring (strict)"("Value"=w367, "Strings []"=w366) -> ()  [unwired: 2 in, 2 out]
              }
              frame "Exposure Priority  **" {
                n241 = call <vilib>:"NT Read String.vi"("Name"=w381) -> ("String"=w380:string)  [unwired: 9 in, 1 out]
                n242 = Index Array(array=w378, index=3) -> (element=w379:cluster{string[]})
                n243 = property on="Test Ring" class="Ring (strict)"("Visible"=TRUE) -> ()  [unwired: 2 in, 2 out]
                n244 = property on="Test Slider" class="Slide (strict)"("Visible"=FALSE) -> ()  [unwired: 2 in, 2 out]
                n245 = Unbundle(w379) -> (w375:string[])
                n246 = Match First String(2:w375, 3:w380) -> (0:w376:i32)  [unwired: 1 out]
                n247 = property on="Test Ring" class="Ring (strict)"("Value"=w376, "Strings []"=w375) -> ()  [unwired: 2 in, 2 out]
              }
              frame "Color Enable  **" {
                n248 = call <vilib>:"NT Read String.vi"("Name"=w390) -> ("String"=w389:string)  [unwired: 9 in, 1 out]
                n249 = Index Array(array=w387, index=4) -> (element=w388:cluster{string[]})
                n250 = property on="Test Ring" class="Ring (strict)"("Visible"=TRUE) -> ()  [unwired: 2 in, 2 out]
                n251 = property on="Test Slider" class="Slide (strict)"("Visible"=FALSE) -> ()  [unwired: 2 in, 2 out]
                n252 = Unbundle(w388) -> (w384:string[])
                n253 = Match First String(2:w384, 3:w389) -> (0:w385:i32)  [unwired: 1 out]
                n254 = property on="Test Ring" class="Ring (strict)"("Value"=w385, "Strings []"=w384) -> ()  [unwired: 2 in, 2 out]
              }
              frame Default {
                n255 = property on="Test Slider" class="Slide (strict)"("Visible"=FALSE) -> ()  [unwired: 2 in, 2 out]
                n256 = property on="Test Ring" class="Ring (strict)"("Visible"=FALSE) -> ()  [unwired: 2 in, 2 out]
              }
              frame "Brightness  **", "Color Level  **", "Compression  **", "FPS  **", "Sharpness  **" {
                n257 = call <vilib>:"NT Read Number.vi"("Name"=w396) -> ("Numeric"=w395:dbl)  [unwired: 9 in, 1 out]
                n258 = property on="Test Ring" class="Ring (strict)"("Visible"=FALSE) -> ()  [unwired: 2 in, 2 out]
                n259 = property on="Test Slider" class="Slide (strict)"("Visible"=TRUE, "Scale.Maximum"=100.0 ("Scale.Range:Maximum")) -> ()  [unwired: 2 in, 2 out]
                n260 = local write "Test Slider"(w395) -> ()
              }
            }
            n261 = property on="Motor" class="Clust (strict)"("Visible"=FALSE) -> ()  [unwired: 2 in, 2 out]
            n262 = property on="On/Off" class="Bool (strict)"("Visible"=FALSE) -> ()  [unwired: 2 in, 2 out]
          }
        }
      }
      event "Test Name": Mouse Enter {
        # "Populate the ring with the list of tests"
        n263 = event-data() -> ()  [unwired: 1 in, 1 out]
        n264 = call <vilib>:"NT Read String Array.vi"("Name"="/TestMode/TestList") -> ("String Array"=w405:string[])  [unwired: 9 in, 1 out]
        n265 = Build Array (concatenate)("Select the test to run...", w405) -> (w404:string[])
        n266 = property on="Test Name" class="Ring (strict)"("Strings []"=w404) -> ()  [unwired: 2 in, 2 out]
      }
      event "Test Name": Value Change {
        w408 = FALSE ("Visible")
        # "Tell the robot the test name to run"
        n267 = event-data() -> ("NewVal"=w412:u16)  [unwired: 1 in]
        n268 = property on="Test Name" class="Ring (strict)"() -> ("Strings []"=w413:string[])  [unwired: 2 in, 2 out]
        n269 = Index Array(array=w413, index=w412) -> (element=w411:string)
        n270 = local write "Progress"(T9 {"Test Progress"=0, "Test Progress Text"=""} ("Progress")) -> ()
        n271 = property on="Progress" class="Clust (strict)"("Visible"=TRUE) -> ()  [unwired: 2 in, 2 out]
        n272 = property on="Test Ring" class="Ring (strict)"("Visible"=w408) -> ()  [unwired: 2 in, 2 out]
        n273 = property on="Motor" class="Clust (strict)"("Visible"=w408) -> ()  [unwired: 2 in, 2 out]
        n274 = property on="Test Slider" class="Slide (strict)"("Visible"=w408) -> ()  [unwired: 2 in, 2 out]
        n275 = property on="On/Off" class="Bool (strict)"("Visible"=w408) -> ()  [unwired: 2 in, 2 out]
        n276 = property on="Rev/Fwd" class="Clust (strict)"("Visible"=w408) -> ()  [unwired: 2 in, 2 out]
        n277 = call <vilib>:"NT Write String.vi"("String"=w411, "Name"="/TestMode/TestName") -> ()  [unwired: 9 in, 1 out]
      }
      event "Command Selection": Value Change {
        # "Get the params and show in table"
        n278 = event-data() -> ("NewVal"=w418:i32)  [unwired: 1 in]
        n279 = property on="Command Selection" class="MCListbox (strict)"() -> ("ItemNames"=w416:string[][])  [unwired: 2 in, 2 out]
        n280 = call <vilib>:"WPI_DashboardUpdate Command Params.vi"("NewVal"=w418, "Commands"=w416, "Param Tbl"=w417) -> ()  [unwired: 8 in, 1 out]
      }
      event "Execute Command": Value Change {
        # "Started one, Unique ID holds\nresponse"
        n281 = event-data() -> ()  [unwired: 1 in, 1 out]
        n282 = property on="Command Selection" class="MCListbox (strict)"() -> ("ItemNames"=w430:string[][])  [unwired: 2 in, 2 out]
        n283 = Index Array(array=w430, index (row)="Command Selection", index (col)=0) -> (element=w428:string)
        n284 = call <vilib>:"Invoke Commands.vi"("Command Params"="Command Params", "Function Name"=w428) -> ("Params"=w424:u8, "Started"=w423:bool)  [unwired: 7 in, 1 out]
        n285 = Array Subset(array="Command Params", length (row)=w424) -> (w425:string[][])  [unwired: 3 in]
        n286 = Select(t="Executing" ("Cmd Status"), s=w423, f="" ("Cmd Status")) -> (s? t:f=→"Cmd Status":string)
      }
      event "Command Selection": Double Click {
        n287 = event-data() -> ("Row"=w440:i32)  [unwired: 1 in]
        n288 = property on="Command Selection" class="MCListbox (strict)"() -> ("ItemNames"=w443:string[][])  [unwired: 2 in, 2 out]
        n289 = local read "Command Params"() -> (w438:string[][])
        n290 = Index Array(array=w443, index (row)=w440, index (col)=0) -> (element=w441:string)
        n291 = call <vilib>:"Invoke Commands.vi"("Command Params"=w438, "Function Name"=w441) -> ("Params"=w437:u8, "Started"=w432:bool)  [unwired: 7 in, 1 out]
        n292 = Array Subset(array=w438, length (row)=w437) -> (w436:string[][])  [unwired: 3 in]
        n293 = Select(t="Executing" ("Cmd Status"), s=w432, f="" ("Cmd Status")) -> (s? t:f=w433:string)
        n294 = local write "Cmd Status"(w433) -> ()
      }
      event "CheckList": Double Click {
        # "Shift clears all"
        # "Update symbols on the listbox"
        n295 = event-data() -> ("PlatMods.Shift"=w446:bool, "Row"=w448:i32)  [unwired: 1 in]
        n296 = case shown="True" w446 {
          tunnel: w448 -> [w452 _]
          tunnel: 1 -> [w451 _]
          frame False {
            n297 = property on="CheckList" class="LstBox (strict)"() -> ("Item Symbols"=w450:i32[])  [unwired: 2 in, 2 out]
            n298 = Replace Array Subset(array=w450, new element=w451, index=w452) -> (w449:i32[])
            n299 = property on="CheckList" class="LstBox (strict)"("Item Symbols"=w449) -> ()  [unwired: 2 in, 2 out]
          }
          frame True {
            w453 = 0 ("Top Row")
            n300 = property on="CheckList" class="LstBox (strict)"() -> ("Number of Rows"=w455:u32)  [unwired: 2 in, 2 out]
            n301 = Initialize Array(0, w455) -> (w454:i32[])
            n302 = property on="CheckList" class="LstBox (strict)"("Top Row"=w453, "Value"=w453, "Item Symbols"=w454) -> ()  [unwired: 2 in, 2 out]
          }
        }
      }
      event "CheckList": Key Down {
        # "Update symbols on the listbox\nLeft and right keys check and uncheck"
        n303 = event-data() -> ("VKey"=w460:T20)  [unwired: 1 in]
        n304 = case shown="\"Left\", \"Right\"" w460 {
          selector: w460 -> [w465 _]
          tunnel: eventvkey."Left" ("VKey") -> [w463 _]
          frame "Left", "Right" {
            n305 = Equal?(x=w463, y=w465) -> (x = y?=w464:bool)
            n306 = Select(t=0, s=w464, f=1) -> (s? t:f=w466:i32)
            n307 = property on="CheckList" class="LstBox (strict)"() -> ("Item Symbols"=w469:i32[])  [unwired: 2 in, 2 out]
            n308 = Replace Array Subset(array=w469, new element=w466, index="CheckList") -> (w468:i32[])
            n309 = property on="CheckList" class="LstBox (strict)"("Item Symbols"=w468) -> ()  [unwired: 2 in, 2 out]
          }
          frame Default {
          }
        }
      }
      event "DB Camera Config": Value Change {
        # "Show or hide the cluster of controls, store in ini file"
        n310 = event-data() -> ("NewVal"=w474:bool)  [unwired: 1 in]
        n311 = case shown="False" w474 {
          tunnel: w473 -> [w483 _]
          tunnel: [w476 w494] -> w472
          tunnel: w471 -> [w475 w494]
          frame False {
            w490 = "Camera"
            w493 = FALSE ("Visible")
            n312 = Index Array(array=w483) -> (element=w486:cluster{string[]})  [unwired: 1 in]
            n313 = local read "Camera Settings"() -> (w482:T4)
            n314 = property on="Camera Settings" class="Clust (strict)"("Visible"=w493) -> ()  [unwired: 2 in, 2 out]
            n315 = local write "DB Camera Config"(w493) -> ()
            n316 = Unbundle(w486) -> (w485:string[])
            n317 = Unbundle(w482) -> ("Frame Rate"=w481:i32, "Compression"=w480:i32, "Size"=w484:u16)
            n318 = Index Array(array=w485, index=w484) -> (element=w479:string)
            n319 = call-poly <vilib>:"Write Key.vi"("section"=w490, "value"=w479, "key"="Size", "refnum"=w475) -> ("refnum out"=w492:T18)  [unwired: 2 in, 5 out]
            n320 = call-poly <vilib>:"Write Key.vi"("section"=w490, "value"=w481, "key"="FrameRate", "refnum"=w492) -> ("refnum out"=w491:T18)  [unwired: 1 in, 6 out]
            n321 = call-poly <vilib>:"Write Key.vi"("section"=w490, "value"=w480, "key"="Compression", "refnum"=w491) -> ("refnum out"=w477:T18)  [unwired: 1 in, 6 out]
            n322 = call <vilib>:"Close Config Data.vi"("refnum"=w477) -> ("file path"=w478:path)  [unwired: 2 in, 8 out]
            n323 = call <vilib>:"Open Config Data.vi"("configuration file path"=w478) -> ("refnum"=w476:T18)  [unwired: 8 in, 2 out]
          }
          frame True {
            n324 = property on="Camera Settings" class="Clust (strict)"("Visible"=TRUE) -> ()  [unwired: 2 in, 2 out]
          }
        }
      }
      event "Camera Settings": Value Change {
        # "Update summary string when any elements of DB camera change"
        n325 = event-data() -> ("NewVal"=w508:T4)  [unwired: 1 in]
        n326 = Index Array(array=w504) -> (element=w503:cluster{string[]})  [unwired: 1 in]
        n327 = Unbundle(w508) -> ("Frame Rate"=w499:i32, "Compression"=w498:i32, "Size"=w501:u16)
        n328 = Unbundle(w503) -> (w502:string[])
        n329 = Index Array(array=w502, index=w501) -> (element=w500:string)
        n330 = Format Into String(format string="%s   %dfps   %d%%", w500, w499, w498) -> (resulting string=w505:string)  [unwired: 2 in, 1 out]
        n331 = Build Array(w505) -> (w506:string[])
        n332 = property on="DB Camera Config" class="Bool (strict)"("Strings [4]"=w506) -> ()  [unwired: 2 in, 2 out]
      }
      event "Motor.Enable": Value Change {
        # "When the test mode otor enable helper is set, update that\ntree row item's value"
        n333 = event-data() -> ("NewVal"=w515:bool)  [unwired: 1 in]
        n334 = Unbundle("Motor") -> ("Value"=w514:dbl)  [unwired: 1 out]
        n335 = Select(t=w514, s=w515, f=0.0) -> (s? t:f=w512:dbl)
        n336 = call <vilib>:"NT Write Number.vi"("Numeric"=w512, "Name"=w511) -> ()  [unwired: 9 in, 1 out]
      }
      event "Test Slider": Value Change {
        # "When the test mode slider helper is set, update that\ntree row item's value"
        n337 = event-data() -> ("NewVal"=w519:dbl)  [unwired: 1 in]
        n338 = call <vilib>:"NT Write Number.vi"("Numeric"=w519, "Name"=w520) -> ()  [unwired: 9 in, 1 out]
      }
      event "On/Off": Value Change {
        # "When the test mode on/off helper value is set, update that\ntree row item's value"
        n339 = event-data() -> ("NewVal"=w525:bool)  [unwired: 1 in]
        n340 = Boolean To (0,1)(Boolean=w525) -> (0, 1=w524:i16)
        n341 = call <vilib>:"NT Write Number.vi"("Numeric"=w524, "Name"=w523) -> ()  [unwired: 9 in, 1 out]
      }
      event "Rev/Fwd": Value Change {
        # "When the test mode helper value for relays is set, update that\ntree row item's value"
        n342 = event-data() -> ("NewVal.Forward"=w534:bool, "NewVal.Reverse"=w533:bool)  [unwired: 1 in]
        n343 = Boolean To (0,1)(Boolean=w534) -> (0, 1=w530:i16)
        n344 = Boolean To (0,1)(Boolean=w533) -> (0, 1=w532:i16)
        n345 = Negate(x=w532) -> (-x=w531:i16)
        n346 = Add(x=w530, y=w531) -> (x+y=w529:i16)
        n347 = call <vilib>:"NT Write Number.vi"("Numeric"=w529, "Name"=w528) -> ()  [unwired: 9 in, 1 out]
      }
      event "Test Ring": Value Change {
        # "When a test mode helper value is selected from the ring,\nset the tree item's variable to the string value"
        n348 = event-data() -> ("NewVal"=w539:u16)  [unwired: 1 in]
        n349 = property on="Test Ring" class="Ring (strict)"() -> ("Strings []"=w540:string[])  [unwired: 2 in, 2 out]
        n350 = Index Array(array=w540, index=w539) -> (element=w538:string)
        n351 = call <vilib>:"NT Write String.vi"("String"=w538, "Name"=w537) -> ()  [unwired: 9 in, 1 out]
      }
      event "Rec Mode": Value Change {
        # "Update globals for recording mode and path to read log from.\nClear when logging and let NetworkTables set path for vision to\nuse."
        n352 = event-data() -> ("NewVal"=w552:enum32{"Stop", "Record", "Playback"})  [unwired: 1 in]
        n353 = global write "WPI_DashboardLogging Global.vi" "Recording"(w552) -> ()
        n354 = case shown="\"Playback\"" w552 {
          tunnel: w551 -> [_ w554 w563]
          tunnel: [_ _ w562] -> w548
          tunnel: [_ _ w561] -> _
          tunnel: w546 -> [_ _ w559]
          tunnel: cluster{i32, i32} {-250, 170} -> [_ _ w558]
          tunnel: [_ _ T21 {"Image Size"=TRUE, "Image Type"=TRUE, "Pixel Value"=TRUE, "ROI Information"=TRUE, "Zoom Factor"=FALSE} ("Image Information Shown:All Elements")] -> w544
          tunnel: [_ _ TRUE ("Zoom Factor")] -> w543
          tunnel: w542 -> [_ _ w555]
          frame Default {
          }
          frame "Stop", "Record" {
            # "Place Window too"
            n355 = invoke class="VI" method="FP.Close"(reference=w554) -> (reference out=w553:refnum<vi>)  [unwired: 2 in, 2 out]
            n356 = invoke class="VI" method="Abort VI"(reference=w553) -> ()  [unwired: 2 in, 3 out]
          }
          frame "Playback" {
            n357 = call "Open Playback Panel.vi"("Offset"=w558, "DB VI Ref"=w559, "Playback in"=w563) -> ("Playback out"=w560:refnum<vi>)  [unwired: 8 in]
            n358 = register-events(w560, w555) -> (reference out=w562:refnum<event-registration>, error out=w561:errorcluster)  [unwired: 2 in]
          }
        }
        n359 = call <vilib>:"WPI_DashboardNT Log FieldName Cache.vi"("Operation"=enum16{"Lookup/Add", "Index", "Clear"}."Clear") -> ()  [unwired: 8 in, 3 out]
        n360 = global write "WPI_DashboardLogging Global.vi" "Logging Filename"(path "") -> ()
        n361 = property on="Camera Image" class="ImageControl"("Image Information Shown"=w544, "Image Information Visible"=w543) -> ()  [unwired: 2 in, 2 out]
      }
      event Panel Close {
        w565 = enum32{"Stop", "Record", "Playback"}."Stop" ("Rec Mode")
        # "Playback window has been closed, abort"
        n362 = event-data() -> ()  [unwired: 1 in, 4 out]
        n363 = local write "Rec Mode"(w565) -> ()
        n364 = global write "WPI_DashboardLogging Global.vi" "Recording"(w565) -> ()
      }
      event Panel Close {
        # "Abort playback window and ourself"
        n365 = event-data() -> ()  [unwired: 1 in, 4 out]
        n366 = invoke class="VI" method="FP.Close"(reference=w571) -> (reference out=w570:refnum<vi>)  [unwired: 2 in, 2 out]
        n367 = invoke class="VI" method="Abort VI"(reference=w570) -> (error out=w569:errorcluster)  [unwired: 2 in, 2 out]
        n368 = invoke class="VI" method="Abort VI"(error in=w569) -> ()  [unwired: 2 in, 3 out]
      }
      event User Event {
        n369 = event-data() -> ("IDs"=w579:cluster{"RPC field ID":u16, "Unique ID":u16}, "String"=w578:string)  [unwired: 1 in]
        n370 = Bundle("IDs"=w579, "String"=w578) -> (w577:T11)  [unwired: 1 in]
        n371 = call <vilib>:"Retrieve RPC Response.vi"("RPC Response"=w577) -> ("Output"=w574:string[][])  [unwired: 10 in]
        n372 = Build Array (concatenate)(w572, w574) -> (w573:string[][])
        n373 = local write "Command Params"(w573) -> ()
        n374 = local write "Cmd Status"("" ("Cmd Status")) -> ()
      }
      event "Vision": Value Change {
        # "Enable/Disable Compression slider.\nHW USB is hard-coded into the camera"
        n375 = event-data() -> ("NewVal"=w586:u16)  [unwired: 1 in]
        n376 = Equal?(x=w586, y=u32 2 ("milliseconds to wait")) -> (x = y?=w584:bool)
        n377 = Select(t=T22."Disabled and Grayed Out" ("Disabled"), s=w584, f=T22."Enabled" ("Disabled")) -> (s? t:f=w581:T22)
        n378 = property on="Compression" class="Slide (strict)"("DisabledEnum"=w581) -> ()  [unwired: 2 in, 2 out]
      }
      event "Tree": Double Click {
        n379 = event-data() -> ("PlatMods"=w591:T25, "Tag"=w590:string)  [unwired: 1 in]
        n380 = Unbundle(w591) -> ("Shift"=w589:bool)  [unwired: 4 out]
        n381 = Not(x=w589) -> (.not. x?=w588:bool)
        n382 = call <vilib>:"NT Update Persistence.vi"("Persistence"=w588, "Name"=w590) -> ()  [unwired: 9 in, 1 out]
      }
    }
  }
  n383 = Tick Count (ms)() -> (millisecond timer value=w1:u32)
  n384 = while {
    tunnel: [w608] -> _
    tunnel: w2 -> [w602]
    tunnel: w15 -> [w601]
    tunnel: w3 -> [w597]
    tunnel: w1 -> [w596]
    shift-right: [w595] -> _
    shift-left: _ -> [w594]
    i -> [w608]
    stop <- FALSE stop-if-true
    n385 = call <vilib>:"WPI_DashboardUpdateNames.vi"("Controls on Tab"=w601) -> ()  [unwired: 11 in]
    n386 = local read "Vision"() -> (w599:u16)
    n387 = call <vilib>:"WPI_DashboardRetrieveStatusInfo.vi"("Vision"=w599, "Binding Refnum"=w602, "Window Mode Notifier"=w597, "TCP Cnx"="TCP") -> ("Power and Errors"=w603:T27, "Robot Metrics"=w606:T28, "Status Info"=w607:T29, "Control Info"=w604:T30, "Robot Mode"=w600:T5, "Process?"=w605:bool)  [unwired: 2 in]
    "Mode" <- w600
    n388 = case shown="True" w605 {
      tunnel: w607 -> [_ w633]
      tunnel: w606 -> [_ w632]
      tunnel: w604 -> [_ w631]
      tunnel: w603 -> [_ w630]
      tunnel: w600 -> [_ _]
      tunnel: w596 -> [_ w614]
      tunnel: [FALSE ("Enabled") w612] -> w595
      tunnel: w594 -> [_ w613]
      frame False {
        (unwired) dbl[] []
        n389 = Wait (ms)(milliseconds to wait=u32 20) -> ()  [unwired: 1 out]
      }
      frame True {
        # "swap motors to match\ncharts and include battery"
        n390 = Unbundle By Name(w632) -> ()  [unwired: 5 out]
        n391 = Unbundle By Name(w630) -> ("Camera Addr"=→"Camera IP":string)  [unwired: 4 out]
        n392 = Unbundle By Name(w631) -> ("Joystick Values"=w627:T31)  [unwired: 5 out]
        n393 = Unbundle By Name(w633) -> ("Status bits"=w615:T32)  [unwired: 1 out]
        n394 = call-poly <vilib>:"NT Read Value.vi"("Name"="RobotDrive Motors") -> ("Numeric Array"=w616:dbl[])  [unwired: 9 in, 1 out]
        n395 = Unbundle By Name(w615) -> ("Enabled"=w612:bool)  [unwired: 7 out]
        n396 = Index Array(array=w616, index #1=1, index #4=0) -> ()  [unwired: 2 in, 4 out]
        n397 = Index Array(array=w627) -> (element #1=w626:T33, element #2=w621:T33)  [unwired: 2 in]
        n398 = case shown="True" w612 {
          tunnel: w614 -> [_ w657]
          tunnel: w613 -> [_ w655]
          tunnel: w612 -> [_ w654]
          frame False {
            n399 = Get Date/Time In Seconds() -> (seconds since 1Jan1904=w646:timestamp)
            n400 = Get Date/Time String(seconds (now)=w646) -> (date string=w644:string, time string=w645:string)  [unwired: 2 in]
            n401 = Search and Replace String(replace all?=TRUE ("replace all? (F)"), input string=w644, search string="/", replace string=" " ("replace string (\"\")")) -> (result string=w637:string)  [unwired: 4 in, 3 out]
            n402 = Search and Replace String(replace all?=TRUE ("replace all? (F)"), input string=w645, search string=":") -> (result string=w635:string)  [unwired: 5 in, 3 out]
            n403 = Concatenate Strings("C:\\frc\\" ("string"), "dlog" ("string"), " " ("string"), w637, " " ("string"), w635, ".txt" ("string")) -> (w649:string)
            n404 = String To Path(string=w649) -> (path=w650:path)
            n405 = String To Path(string="C:\\frc\\templog.txt") -> (path=w651:path)
            n406 = Copy(10:w650, 11:w651) -> (0:w652:errorcluster)  [unwired: 3 in, 2 out]
            n407 = Delete(path (use dialog)=w651, error in=w652) -> ()  [unwired: 3 in, 3 out]
          }
          frame True {
            n408 = Not Equal?(x=w654, y=w655) -> (x != y?=w656:bool)
            n409 = case shown="False" w656 {
              tunnel: w657 -> [w766 _]
              frame False {
                w661 = "\t" ("string")
                # "Remove"
                # "Remove"
                # "Remove"
                # "Remove"
                n410 = Tick Count (ms)() -> (millisecond timer value=w768:u32)
                n411 = Subtract(x=w768, y=w766) -> (x-y=w767:u32)
                n412 = call-poly <vilib>:"NT Read Value.vi"("Name"="Arm Encoder Position") -> ("Numeric"=w762:dbl)  [unwired: 9 in, 1 out]
                "Arm Encoder" <- w762
                n413 = call-poly <vilib>:"NT Read Value.vi"("Name"="Shooter Current") -> ("Numeric"=w705:dbl)  [unwired: 9 in, 1 out]
                "Shooter Current" <- w705
                n414 = local read "Target Distance"() -> (w765:dbl)
                n415 = String To Path(string="C:\\frc\\templog.txt") -> (path=w778:path)
                n416 = call-poly <vilib>:"NT Read Value.vi"("Name"="At Target") -> ("Boolean"=w659:bool)  [unwired: 9 in, 1 out]
                n417 = call-poly <vilib>:"NT Read Value.vi"("Name"="Angle At Setpoint") -> ("Boolean"=w667:bool)  [unwired: 9 in, 1 out]
                n418 = call-poly <vilib>:"NT Read Value.vi"("Name"="Angle Is Enabled") -> ("Boolean"=w665:bool)  [unwired: 9 in, 1 out]
                n419 = call-poly <vilib>:"NT Read Value.vi"("Name"="Arm PID At SetPoint") -> ("Boolean"=w747:bool)  [unwired: 9 in, 1 out]
                n420 = call-poly <vilib>:"NT Read Value.vi"("Name"="Auton Finished") -> ("Boolean"=w730:bool)  [unwired: 9 in, 1 out]
                n421 = call-poly <vilib>:"NT Read Value.vi"("Name"="Auton Shooting Or Not") -> ("Boolean"=w715:bool)  [unwired: 9 in, 1 out]
                n422 = call-poly <vilib>:"NT Read Value.vi"("Name"="Gear Shift Current") -> ("Numeric"=w706:dbl)  [unwired: 9 in, 1 out]
                n423 = call-poly <vilib>:"NT Read Value.vi"("Name"="Total Current") -> ("Numeric"=w686:dbl)  [unwired: 9 in, 1 out]
                n424 = call-poly <vilib>:"NT Read Value.vi"("Name"="Right Lift Current") -> ("Numeric"=w689:dbl)  [unwired: 9 in, 1 out]
                n425 = call-poly <vilib>:"NT Read Value.vi"("Name"="ANGLE") -> ("Numeric"=w672:dbl)  [unwired: 9 in, 1 out]
                n426 = call-poly <vilib>:"NT Read Value.vi"("Name"="Angle PID Point") -> ("Numeric"=w669:dbl)  [unwired: 9 in, 1 out]
                n427 = call-poly <vilib>:"NT Read Value.vi"("Name"="Left Lift Current") -> ("Numeric"=w691:dbl)  [unwired: 9 in, 1 out]
                n428 = call-poly <vilib>:"NT Read Value.vi"("Name"="Roller Current") -> ("Numeric"=w693:dbl)  [unwired: 9 in, 1 out]
                n429 = call-poly <vilib>:"NT Read Value.vi"("Name"="Right Pivot Current") -> ("Numeric"=w695:dbl)  [unwired: 9 in, 1 out]
                n430 = call-poly <vilib>:"NT Read Value.vi"("Name"="Left Pivot Current") -> ("Numeric"=w697:dbl)  [unwired: 9 in, 1 out]
                n431 = call-poly <vilib>:"NT Read Value.vi"("Name"="Right Drive Rear Current") -> ("Numeric"=w699:dbl)  [unwired: 9 in, 1 out]
                n432 = call-poly <vilib>:"NT Read Value.vi"("Name"="Right Drive Front Current") -> ("Numeric"=w701:dbl)  [unwired: 9 in, 1 out]
                n433 = call-poly <vilib>:"NT Read Value.vi"("Name"="Left Drive Rear Current") -> ("Numeric"=w684:dbl)  [unwired: 9 in, 1 out]
                n434 = call-poly <vilib>:"NT Read Value.vi"("Name"="Left Drive Front Current") -> ("Numeric"=w685:dbl)  [unwired: 9 in, 1 out]
                n435 = call-poly <vilib>:"NT Read Value.vi"("Name"="Screw Encoder Position") -> ("Numeric"=w757:dbl)  [unwired: 9 in, 1 out]
                n436 = call-poly <vilib>:"NT Read Value.vi"("Name"="Arm Right Encoder Position") -> ("Numeric"=w755:dbl)  [unwired: 9 in, 1 out]
                n437 = call-poly <vilib>:"NT Read Value.vi"("Name"="Screw Right Encoder Position") -> ("Numeric"=w751:dbl)  [unwired: 9 in, 1 out]
                n438 = call-poly <vilib>:"NT Read Value.vi"("Name"="Arm PID SetPoint") -> ("Numeric"=w759:dbl)  [unwired: 9 in, 1 out]
                n439 = call-poly <vilib>:"NT Read Value.vi"("Name"="Shooter Status") -> ("Numeric"=w745:dbl)  [unwired: 9 in, 1 out]
                n440 = call-poly <vilib>:"NT Read Value.vi"("Name"="Drive Encoder Distance") -> ("Numeric"=w743:dbl)  [unwired: 9 in, 1 out]
                n441 = call-poly <vilib>:"NT Read Value.vi"("Name"="Drive Left Encoder Distance") -> ("Numeric"=w681:dbl)  [unwired: 9 in, 1 out]
                n442 = call-poly <vilib>:"NT Read Value.vi"("Name"="Drive Right Encoder Distance") -> ("Numeric"=w679:dbl)  [unwired: 9 in, 1 out]
                n443 = call-poly <vilib>:"NT Read Value.vi"("Name"="Drive Average Speed") -> ("Numeric"=w739:dbl)  [unwired: 9 in, 1 out]
                n444 = call-poly <vilib>:"NT Read Value.vi"("Name"="Drive Left Speed") -> ("Numeric"=w675:dbl)  [unwired: 9 in, 1 out]
                n445 = call-poly <vilib>:"NT Read Value.vi"("Name"="Drive Right Speed") -> ("Numeric"=w677:dbl)  [unwired: 9 in, 1 out]
                n446 = call-poly <vilib>:"NT Read Value.vi"("Name"="Auton Case") -> ("Numeric"=w732:dbl)  [unwired: 9 in, 1 out]
                n447 = call-poly <vilib>:"NT Read Value.vi"("Name"="Auton Timer") -> ("Numeric"=w726:dbl)  [unwired: 9 in, 1 out]
                n448 = call-poly <vilib>:"NT Read Value.vi"("Name"="Shooter Left Talon") -> ("Numeric"=w723:dbl)  [unwired: 9 in, 1 out]
                n449 = call-poly <vilib>:"NT Read Value.vi"("Name"="Shooter Right Talon") -> ("Numeric"=w721:dbl)  [unwired: 9 in, 1 out]
                n450 = call-poly <vilib>:"NT Read Value.vi"("Name"="Auton Defense Location") -> ("Numeric"=w717:dbl)  [unwired: 9 in, 1 out]
                n451 = call-poly <vilib>:"NT Read Value.vi"("Name"="Auton Defense Type") -> ("Numeric"=w719:dbl)  [unwired: 9 in, 1 out]
                n452 = local read "Target X"() -> (w764:dbl)
                n453 = local read "Target Y"() -> (w763:dbl)
                n454 = Divide(x=w767, y=u32 1000) -> (x/y=w782:dbl)
                n455 = Format Into String(w764) -> (resulting string=w791:string)  [unwired: 3 in, 1 out]
                n456 = Format Into String(w763) -> (resulting string=w792:string)  [unwired: 3 in, 1 out]
                n457 = Format Into String(w762) -> (resulting string=w761:string)  [unwired: 3 in, 1 out]
                n458 = Format Into String(w706) -> (resulting string=w793:string)  [unwired: 3 in, 1 out]
                n459 = Format Into String(w782) -> (resulting string=w790:string)  [unwired: 3 in, 1 out]
                n460 = Format Into String(w659) -> (resulting string=w658:string)  [unwired: 3 in, 1 out]
                n461 = Format Into String(w686) -> (resulting string=w794:string)  [unwired: 3 in, 1 out]
                n462 = Format Into String(w705) -> (resulting string=w784:string)  [unwired: 3 in, 1 out]
                n463 = Format Into String(w689) -> (resulting string=w797:string)  [unwired: 3 in, 1 out]
                n464 = Format Into String(w672) -> (resulting string=w671:string)  [unwired: 3 in, 1 out]
                n465 = Format Into String(w669) -> (resulting string=w664:string)  [unwired: 3 in, 1 out]
                n466 = Format Into String(w667) -> (resulting string=w663:string)  [unwired: 3 in, 1 out]
                n467 = Format Into String(w665) -> (resulting string=w662:string)  [unwired: 3 in, 1 out]
                n468 = Format Into String(w765) -> (resulting string=w783:string)  [unwired: 3 in, 1 out]
                n469 = Format Into String(w691) -> (resulting string=w795:string)  [unwired: 3 in, 1 out]
                n470 = Format Into String(w693) -> (resulting string=w796:string)  [unwired: 3 in, 1 out]
                n471 = Format Into String(w695) -> (resulting string=w785:string)  [unwired: 3 in, 1 out]
                n472 = Format Into String(w697) -> (resulting string=w786:string)  [unwired: 3 in, 1 out]
                n473 = Format Into String(w699) -> (resulting string=w787:string)  [unwired: 3 in, 1 out]
                n474 = Format Into String(w701) -> (resulting string=w788:string)  [unwired: 3 in, 1 out]
                n475 = Format Into String(w684) -> (resulting string=w708:string)  [unwired: 3 in, 1 out]
                n476 = Format Into String(w685) -> (resulting string=w760:string)  [unwired: 3 in, 1 out]
                n477 = Format Into String(w757) -> (resulting string=w753:string)  [unwired: 3 in, 1 out]
                n478 = Format Into String(w755) -> (resulting string=w752:string)  [unwired: 3 in, 1 out]
                n479 = Format Into String(w751) -> (resulting string=w749:string)  [unwired: 3 in, 1 out]
                n480 = Format Into String(w759) -> (resulting string=w748:string)  [unwired: 3 in, 1 out]
                n481 = Format Into String(w747) -> (resulting string=w741:string)  [unwired: 3 in, 1 out]
                n482 = Format Into String(w745) -> (resulting string=w740:string)  [unwired: 3 in, 1 out]
                n483 = Format Into String(w743) -> (resulting string=w683:string)  [unwired: 3 in, 1 out]
                n484 = Format Into String(w681) -> (resulting string=w737:string)  [unwired: 3 in, 1 out]
                n485 = Format Into String(w679) -> (resulting string=w682:string)  [unwired: 3 in, 1 out]
                n486 = Format Into String(w739) -> (resulting string=w736:string)  [unwired: 3 in, 1 out]
                n487 = Format Into String(w675) -> (resulting string=w735:string)  [unwired: 3 in, 1 out]
                n488 = Format Into String(w677) -> (resulting string=w734:string)  [unwired: 3 in, 1 out]
                n489 = Format Into String(w732) -> (resulting string=w728:string)  [unwired: 3 in, 1 out]
                n490 = Format Into String(w730) -> (resulting string=w727:string)  [unwired: 3 in, 1 out]
                n491 = Format Into String(w726) -> (resulting string=w724:string)  [unwired: 3 in, 1 out]
                n492 = Format Into String(w723) -> (resulting string=w713:string)  [unwired: 3 in, 1 out]
                n493 = Format Into String(w721) -> (resulting string=w712:string)  [unwired: 3 in, 1 out]
                n494 = Format Into String(w717) -> (resulting string=w711:string)  [unwired: 3 in, 1 out]
                n495 = Format Into String(w719) -> (resulting string=w710:string)  [unwired: 3 in, 1 out]
                n496 = Format Into String(w715) -> (resulting string=w709:string)  [unwired: 3 in, 1 out]
                n497 = call <vilib>:"Open_Create_Replace File.vi"("function (open:0)"=T26."open or create", "file path"=w778) -> ("error out"=w770:errorcluster, "file size (bytes)"=w772:i32, "refnum"=w771:refnum<file>)  [unwired: 6 in, 1 out]
                n498 = Concatenate Strings(w790, w661, w658, w661, w671, w661, w664, w661, w663, w661, w662, w661, w783, w661, w791, w661, w792, w661, w761, w661, w793, w661, w794, w661, w784, w661, w797, w661, w795, w661, w796, w661, w785, w661, w786, w661, w787, w661, w788, w661, w708, w661, w760, w661, w753, w661, w752, w661, w749, w661, w748, w661, w741, w661, w740, w661, w683, w661, w737, w661, w682, w661, w736, w661, w735, w661, w734, w661, w728, w661, w727, w661, w724, w661, w713, w661, w712, w661, w711, w661, w710, w661, w709, "\n" ("string")) -> (w780:string)
                n499 = Set File Position(offset (in bytes) (0)=w772, refnum=w771, error in=w770) -> (refnum out=w775:refnum<file>, error out=w776:errorcluster)  [unwired: 1 in]
                n500 = Write to Binary File(file (use dialog)=w775, data=w780, error in=w776, 5:FALSE ("prepend array or string size? (T)")) -> (refnum out=w774:refnum<file>, error out=w773:errorcluster)  [unwired: 2 in, 1 out]
                n501 = Close File(refnum=w774, error in=w773) -> ()  [unwired: 2 out]
              }
              frame True {
                w799 = "\t" ("string")
                n502 = String To Path(string="C:\\frc\\templog.txt") -> (path=w845:path)
                n503 = call <vilib>:"Open_Create_Replace File.vi"("function (open:0)"=T26."open or create", "file path"=w845) -> ("error out"=w853:errorcluster, "file size (bytes)"=w851:i32, "refnum"=w852:refnum<file>)  [unwired: 6 in, 1 out]
                n504 = Set File Position(offset (in bytes) (0)=w851, refnum=w852, error in=w853) -> (refnum out=w848:refnum<file>, error out=w847:errorcluster)  [unwired: 1 in]
                n505 = Concatenate Strings("time" ("string"), w799, "At Taget", w799, "ANGLE", w799, "Angle PID Point", w799, "Angle At Setpoint", w799, "Angle Is Enabled", w799, "Distance" ("string"), w799, "Camera X" ("string"), w799, "Camera Y" ("string"), w799, "Arm Encoder" ("string"), w799, "Left Front Drive Current" ("string"), w799, "Left Rear Drive Current" ("string"), w799, "Right Front Drive Current" ("string"), w799, "Right Rear Drive Current" ("string"), w799, "Pivot Left Current" ("string"), w799, "Pivot Right Current" ("string"), w799, "Roller Current" ("string"), w799, "Lift Left Current" ("string"), w799, "Lift Right Current" ("string"), w799, "Shoot Current" ("string"), w799, "Gear Shift Current", w799, "Total Current" ("string"), w799, "Screw Encoder Position", w799, "Arm Right Encoder Position", w799, "Screw Right Encoder Position", w799, "Arm PID SetPoint", w799, "Arm PID At SetPoint", w799, "Shooter Status", w799, "Drive Encoder Distance", w799, "dDrive Left Encoder Distance", w799, "dDrive Right Encoder Distatnce", w799, "Drive Average Speed", w799, "dDrive Left Speed", w799, "dDrive Right Speed", w799, "Auton Case", w799, "Auton Finished", w799, "Auton Timer", w799, "Shooter Left Talon", w799, "Shooter Right Talon", w799, "Auton Defense Location", w799, "Auton Defense Type", w799, "Auton Shooting Or Not", "\n" ("string")) -> (w827:string)
                n506 = Write to Binary File(file (use dialog)=w848, data=w827, error in=w847, 5:FALSE ("prepend array or string size? (T)")) -> (refnum out=w849:refnum<file>, error out=w850:errorcluster)  [unwired: 2 in, 1 out]
                n507 = Close File(refnum=w849, error in=w850) -> ()  [unwired: 2 out]
              }
            }
          }
        }
        n508 = call "Prepare Joystick Data for Displays.vi"("Joystick Values"=w626) -> ("Buttons"=→"JS1 Buttons":T34, "Z Axis"=→"JS1 Z":dbl, "Cartesian Data"=→"JS1 Graph":cluster{"X axis":dbl, "X axis":dbl}[])  [unwired: 8 in]
        n509 = call "Prepare Joystick Data for Displays.vi"("Joystick Values"=w621) -> ("Buttons"=→"JS2 Buttons":T34, "Z Axis"=→"JS2 Z":dbl, "Cartesian Data"=→"JS2 Graph":cluster{"X axis":dbl, "X axis":dbl}[])  [unwired: 8 in]
      }
    }
  }
